vi "pyonpyon3.7.vi"() -> ()   [LabVIEW 2013]
uses:
  impl/CTL_pp3c_SessionParam.ctl
  impl/pp3_CTL_SessionInfo.ctl
  impl/CTL_pp3g_LoopState.ctl
  impl/pp3_CTL_BehavioralState.ctl
  impl/CTL_pp3g_Trial.ctl
  impl/pp3_CTL_TrialType.ctl
  labolabo2/waveforms/WFTypes.ctl
  impl/pp3_CTL_SessionParamDynamic.ctl
  impl/CTL_pp3c_DaqStatus.ctl
  <vilib>/userdefined/High Color/IMAQdx.ctl
  <vilib>/sound2/lvsound2.llb/Sound Output Task ID.ctl
  labolabo2/array/impl/NullArray_I.vi
  <vilib>/Utility/file.llb/Read From Spreadsheet File (string).vi
  labolabo2/array/impl/ArrayFirst_S.vi
panel:
  out "Session List Valid":bool=TRUE
  in  "Refresh info":bool
  in  "Session List Hidden":u8[](array[numeric])=[1, 1, 1, 2, 2, 2, 1, 1, 2, 2, 2, 1, 2, 1, 2, 2, 1, 1, 2, 2, 2, 1, 1, 1, 2, 2, 2, 1, 2, 1, 2, 1, 2, 1, 1, 1, 2, 2, 1, 2, 1, 1, 2, 1, 2, 1, 2, 1, 2, 2, 2, 1, 2, 1, 2, 1, 2, 1, 1, 1] min=1 step=1
  out "concatenated string":string="OS Name:                   Microsoft Wi\rOS Version:                6.1.7601 Service Pack 1 Build 7601\rSystem Type:               x64-based PC\rTime Zone:                 (UTC+01:00) Amsterdam, Berli\rTotal Physical Memory:     7,657 MB"
  out "Info VI Revision":string="1403" caption="Rev #"
  out "Info Hostname":string="PCR6985-17"
  out "Session list display":string[][](table)=[["1", "1", "1", "2", "2"], ["2", "1", "1", "2", "2"], ["2", "1", "2", "1", "2"], ["2", "1", "1", "2", "2"], ["2", "1", "1", "1", "2"], ["2", "2", "1", "2", "1"], ["2", "1", "2", "1", "1"], ["1", "2", "2", "1", "2"], ["1", "1", "2", "1", "2"], ["1", "2", "1", "2", "2"], ["2", "1", "2", "1", "2"], ["1", "2", "1", "1", "1"]]
  in  "Trial Types Control":enum32{"Trial Types Control"}(tab)
  out "Trial Types File Path":path=path "C:/Data/tDC.Coulb2/trial types/01_02__FM2k4k_4k2k.pp2tt.tsv"
  in  "Save Trial Types":bool
  in  "Load Trial Types":bool
  out "Trial Types Valid":bool=TRUE
  in  "Trial Types":T1[](array[typedef])=[{"Trial Type Number"=1, "Trial Type"=enum."GO", "Trial Weight"=1, "Shock (mA)"=-1.0, "Duration (ms)"=250.0, "Sound Type"=enum."04 FM Sweep", "Stim P1"=2000.0, "Stim P2"=4000.0, "Stim P3"=0.0, "Stim P4"=0.0, "DAQ Amplitude (V)"=1.0}, {"Trial Type Number"=2, "Trial Type"=enum."NOGO", "Trial Weight"=1, "Shock (mA)"=-1.0, "Duration (ms)"=250.0, "Sound Type"=enum."04 FM Sweep", "Stim P1"=4000.0, "Stim P2"=2000.0, "Stim P3"=0.0, "Stim P4"=0.0, "DAQ Amplitude (V)"=1.0}] {"DAQ Amplitude (V)" min=0.0 max=5.0 format="%_4g"; "Shock (mA)" min=-1.0 max=5.0; "Trial Weight" step=1; "Duration (ms)" min=0.0 max=1.0; "Trial Type Number" min=1 max=256 step=1}
  in  "Session List Control":enum32{"Session List Control"}(tab)
  out "Session List File Path":path
  in  "Load Session List":bool
  in  "Save Session List":bool
  in  "Generate Session List":bool
  in  "Total Trials":i32=60 min=3 max=122 step=1
  in  "Pseudo-Gell. Start":i32=2 min=0 max=3 step=1
  in  "60 trials":bool
  in  "90 trials":bool
  in  "test trials":bool
  in  "DAQ status variable":T4={"Sound AO"="Dev6/ao0", "Shock intesity AO"="Dev6/ao1", "Code_LED DO"="Dev6/port1:2", "Switch DI"="Dev6/port0/line0", "Webcam"="cam9", "Sound AO task"="", "Sound card task"=0, "Shock intensity AO task"="", "Code_LED DO task"="", "Switch DI task"="", "AO <=> Sound card"=FALSE, "Sound card"=0, "sample rate"=100000.0, "Variable shock"=TRUE, "Webcam on"=TRUE, "Waveform memo"={"t0"=timestamp(0 s since 1904-01-01), "dt"=1.0, "Y"=[]}, "Tone trigger"="PFI1", "Master-9 DO"="Dev6/port0/line5:7", "Master-9 DO task"="", "Master-9 on"=TRUE} caption="DAQ status variable  (initially to be read from /config/config.main.vi, change default settings there)" {"sample rate" min=8000.0; "Sound card task" format="%.0x"}
  out "Image":T7(plugin-control)
  in  "Session param (dynamic)":T8={"Def M shock (uA)"=720.0, "Def F shock (uA)"=150.0}
  in  "stop":bool
  in  "Pause":bool
  out "Loop state":T9={"Curr  tr"=2, "Curr (ms)"=2873456, "Cum (ms)"=46921, "Run loop diff"=11, "Tone countdown (ms)"=777777, "Countdown (ms)"=764, "Curr State"=enum."14 Intertrial Interval", "Prev State"=enum."9 NOGO Jumped", "Rw"=FALSE, "Sw"=FALSE, "Tone\nGate"=FALSE, "Punish"=FALSE, "Current DAQ DO Int"=0, "Current Loaded Trial"={"Trial Type Number"=2, "Trial Type"=enum."NOGO", "Trial Weight"=1, "Shock (mA)"=150.0, "Duration (ms)"=250.0, "Sound Type"=enum."04 FM Sweep", "Stim P1"=4000.0, "Stim P2"=2000.0, "Stim P3"=0.0, "Stim P4"=0.0, "DAQ Amplitude (V)"=1.0}, "Total trials memo"=60, "State start cum memo (ms)"=42685, "Last dur jump time memo (ms)"=1563, "Last dur shock time memo (ms)"=3019, "Tone repeat memo (ms)"=0, "Webcam on"=FALSE, "Webcam recording"=FALSE, "State update flag"=FALSE, "Last loaded shock voltage"=0.075, "Vid upd"=enum."0", "First time tone"=FALSE} {"Current DAQ DO Int" format="%016b"; "Current Loaded Trial"."DAQ Amplitude (V)" min=0.0 max=5.0 format="%_4g"; "Current Loaded Trial"."Shock (mA)" min=-1.0 max=5.0; "Current Loaded Trial"."Trial Weight" step=1; "Current Loaded Trial"."Duration (ms)" min=0.0 max=1.0; "Current Loaded Trial"."Trial Type Number" min=1 max=256 step=1}
  in  "Session parameters":T11={"Log File Directory Root"=path "E:/Data/SPP.Coulb1", "Subject Name"="test", "Tone repeat (ms)"=0, "Habit tr0 (s)"=180, "ITI min\n(s)"=14, "ITI max\n(s)"=24, "Stay \n(s)"=5, "Run"=FALSE, "Jump time\n(s)"=4, "Start trial"=0, "Log File Directory"=path "C:/Data/tDC.Coulb2/test/171120/163328", "Shock \ndur (s)"=6, "Pre click \n(V)"=0.1, "Click\ndel (s)"=1.0, "Reward CR"=FALSE} {"Click\ndel (s)" min=0.0 step=1.0; "Pre click \n(V)" min=0.0 max=1.0 step=1.0; "Shock \ndur (s)" min=0 step=1; "Stay \n(s)" min=0 step=1; "Start trial" step=1; "Jump time\n(s)" min=0 step=1; "Tone repeat (ms)" min=0 max=1000 step=1; "ITI min\n(s)" min=0 step=1; "ITI max\n(s)" min=0 step=1; "Habit tr0 (s)" min=0 step=1}
  out "Runtime Errors":errorcluster
  in  "Refresh":bool
  out "Session info":T12={"Total  Tr"=3, "G Tr"=2, "G Jump"=0, "G Jump%"=0.0, "N Tr"=1, "N Jump"=1, "N Jump%"=100.0, "T Tr"=0, "T Jump"=0, "T Jump%"=nan, "M shock dur (ms)"=1503.5, "F shock dur (ms)"=3019.0, "H latency (ms)"=0.0, "F latency (ms)"=1563.0, "T jump latency (ms)"=0.0} {"T Jump%" format="%.3g"; "N Jump%" format="%.3g"; "G Jump%" format="%.3g"}
  # "Pyonpyon Labview  v3.7 \n(2017.3 KT -- opto trig C)"
  # "60 trials:  180-14-24-5\n90 trials:  180-6-16-3"
  # "Code"
  # "Type"
  # "P 1"
  # "P 2"
  # "P 3"
  # "P 4 (opto)"
  # "Weight"
  # "Shock"
  # "Dur (ms)"
  # "DAQ Ampl (V)"
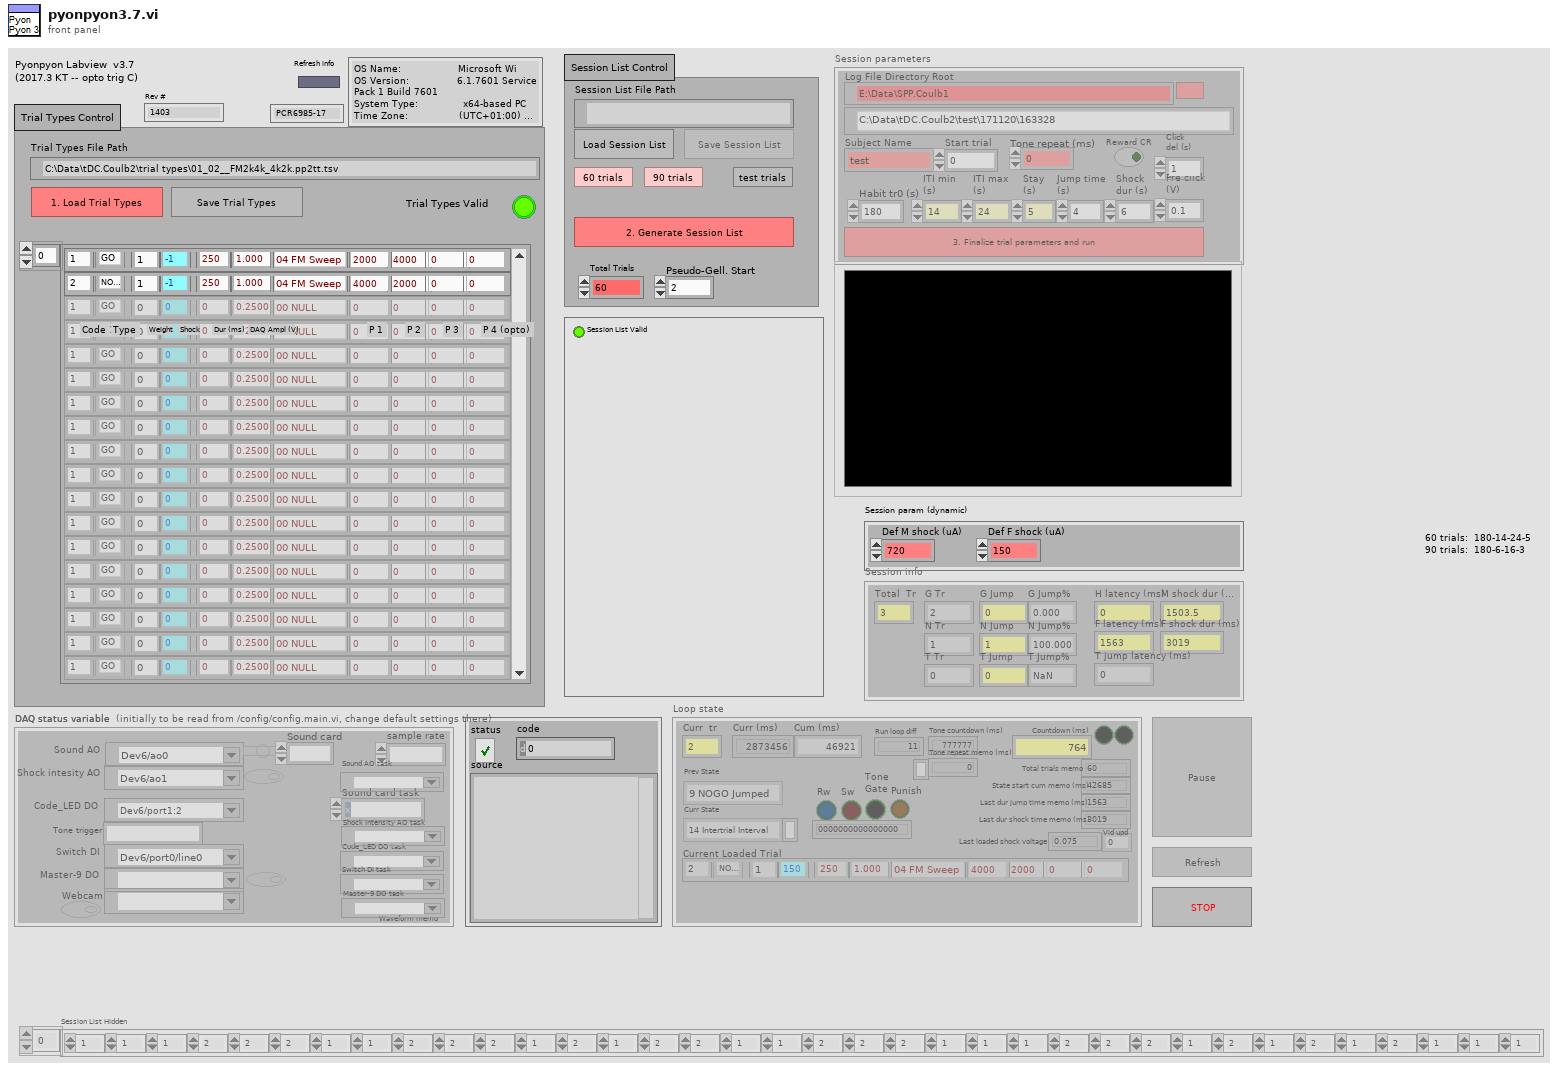
[diagram p1: front panel]
types:
  T1 = typedef "CTL_pp3g_Trial.ctl" = cluster{"Trial Type Number":i16, "Trial Type":T2, "Trial Weight":u32, "Shock (mA)":dbl, "Duration (ms)":dbl, "Sound Type":T3, "Stim P1":dbl, "Stim P2":dbl, "Stim P3":dbl, "Stim P4":dbl, "DAQ Amplitude (V)":dbl}
  T2 = typedef "pp3_CTL_TrialType.ctl" = enum16{"OFF", "GO", "NOGO", "TEST"}
  T3 = typedef "WFTypes.ctl" = enum16{"00 NULL", "01 DC", "02 Noise", "03 Pure Tone", "04 FM Sweep", "05 FM Sweep BURST"}
  T4 = typedef "CTL_pp3c_DaqStatus.ctl" = cluster{"Sound AO":tag, "Shock intesity AO":tag, "Code_LED DO":tag, "Switch DI":tag, "Webcam":T5, "Sound AO task":refnum<k21>, "Sound card task":T6, "Shock intensity AO task":refnum<k21>, "Code_LED DO task":refnum<k21>, "Switch DI task":refnum<k21>, "AO <=> Sound card":bool, "Sound card":u32, "sample rate":dbl, "Variable shock":bool, "Webcam on":bool, "Waveform memo":waveform(dbl), "Tone trigger":string, "Master-9 DO":tag, "Master-9 DO task":refnum<k21>, "Master-9 on":bool}
  T5 = typedef "IMAQdx.ctl" = refnum<k21>
  T6 = typedef "Sound Output Task ID.ctl" = u32
  T7 = typedef "IMAQ Image.ctl" = refnum<image>
  T8 = typedef "pp3_CTL_SessionParamDynamic.ctl" = cluster{"Def M shock (uA)":dbl, "Def F shock (uA)":dbl}
  T9 = typedef "CTL_pp3g_LoopState.ctl" = cluster{"Curr  tr":u16, "Curr (ms)":u32, "Cum (ms)":u64, "Run loop diff":i64, "Tone countdown (ms)":i64, "Countdown (ms)":i64, "Curr State":T10, "Prev State":T10, "Rw":bool, "Sw":bool, "Tone\nGate":bool, "Punish":bool, "Current DAQ DO Int":u16, "Current Loaded Trial":T1, "Total trials memo":i64, "State start cum memo (ms)":i64, "Last dur jump time memo (ms)":i64, "Last dur shock time memo (ms)":i64, "Tone repeat memo (ms)":i64, "Webcam on":bool, "Webcam recording":bool, "State update flag":bool, "Last loaded shock voltage":dbl, "Vid upd":enum16{"0", "1", "2", "3", "4", "5", "6", "7", "8", "9"}, "First time tone":bool}
  T10 = typedef "pp3_CTL_BehavioralState.ctl" = enum8{"0 NULL", "1 Habituation", "2 (Load Trial)", "3 Stay Period", "4 Load Audio/Click Delay", "5 GO Trial", "6 GO Jumped", "7 GO Timeout", "8 NOGO Trial", "9 NOGO Jumped", "10 NOGO Timeout", "11 TEST Trial", "12 TEST Jumped", "13 TEST Timeout", "14 Intertrial Interval", "15 Done"}
  T11 = typedef "CTL_pp3c_SessionParam.ctl" = cluster{"Log File Directory Root":path, "Subject Name":string, "Tone repeat (ms)":i32, "Habit tr0 (s)":i32, "ITI min\n(s)":i32, "ITI max\n(s)":i32, "Stay \n(s)":i32, "Run":bool, "Jump time\n(s)":i32, "Start trial":u16, "Log File Directory":path, "Shock \ndur (s)":i32, "Pre click \n(V)":dbl, "Click\ndel (s)":dbl, "Reward CR":bool}
  T12 = typedef "pp3_CTL_SessionInfo.ctl" = cluster{"Total  Tr":u32, "G Tr":u32, "G Jump":u32, "G Jump%":dbl, "N Tr":u32, "N Jump":u32, "N Jump%":dbl, "T Tr":u32, "T Jump":u32, "T Jump%":dbl, "M shock dur (ms)":dbl, "F shock dur (ms)":dbl, "H latency (ms)":dbl, "F latency (ms)":dbl, "T jump latency (ms)":dbl}
  T13 = enum8{"Enabled", "Disabled", "Disabled and Grayed Out"}
  T14 = enum16{"open", "replace", "create", "open or create", "replace or create", "replace or create with confirmation"}
  T15 = typedef "imagedata.ctl" = cluster{"image type":i32, "image depth":i32, "image":u8[], "mask":u8[], "colors":u32[], "Rectangle":cluster{"left":i16, "top":i16, "right":i16, "bottom":i16}}
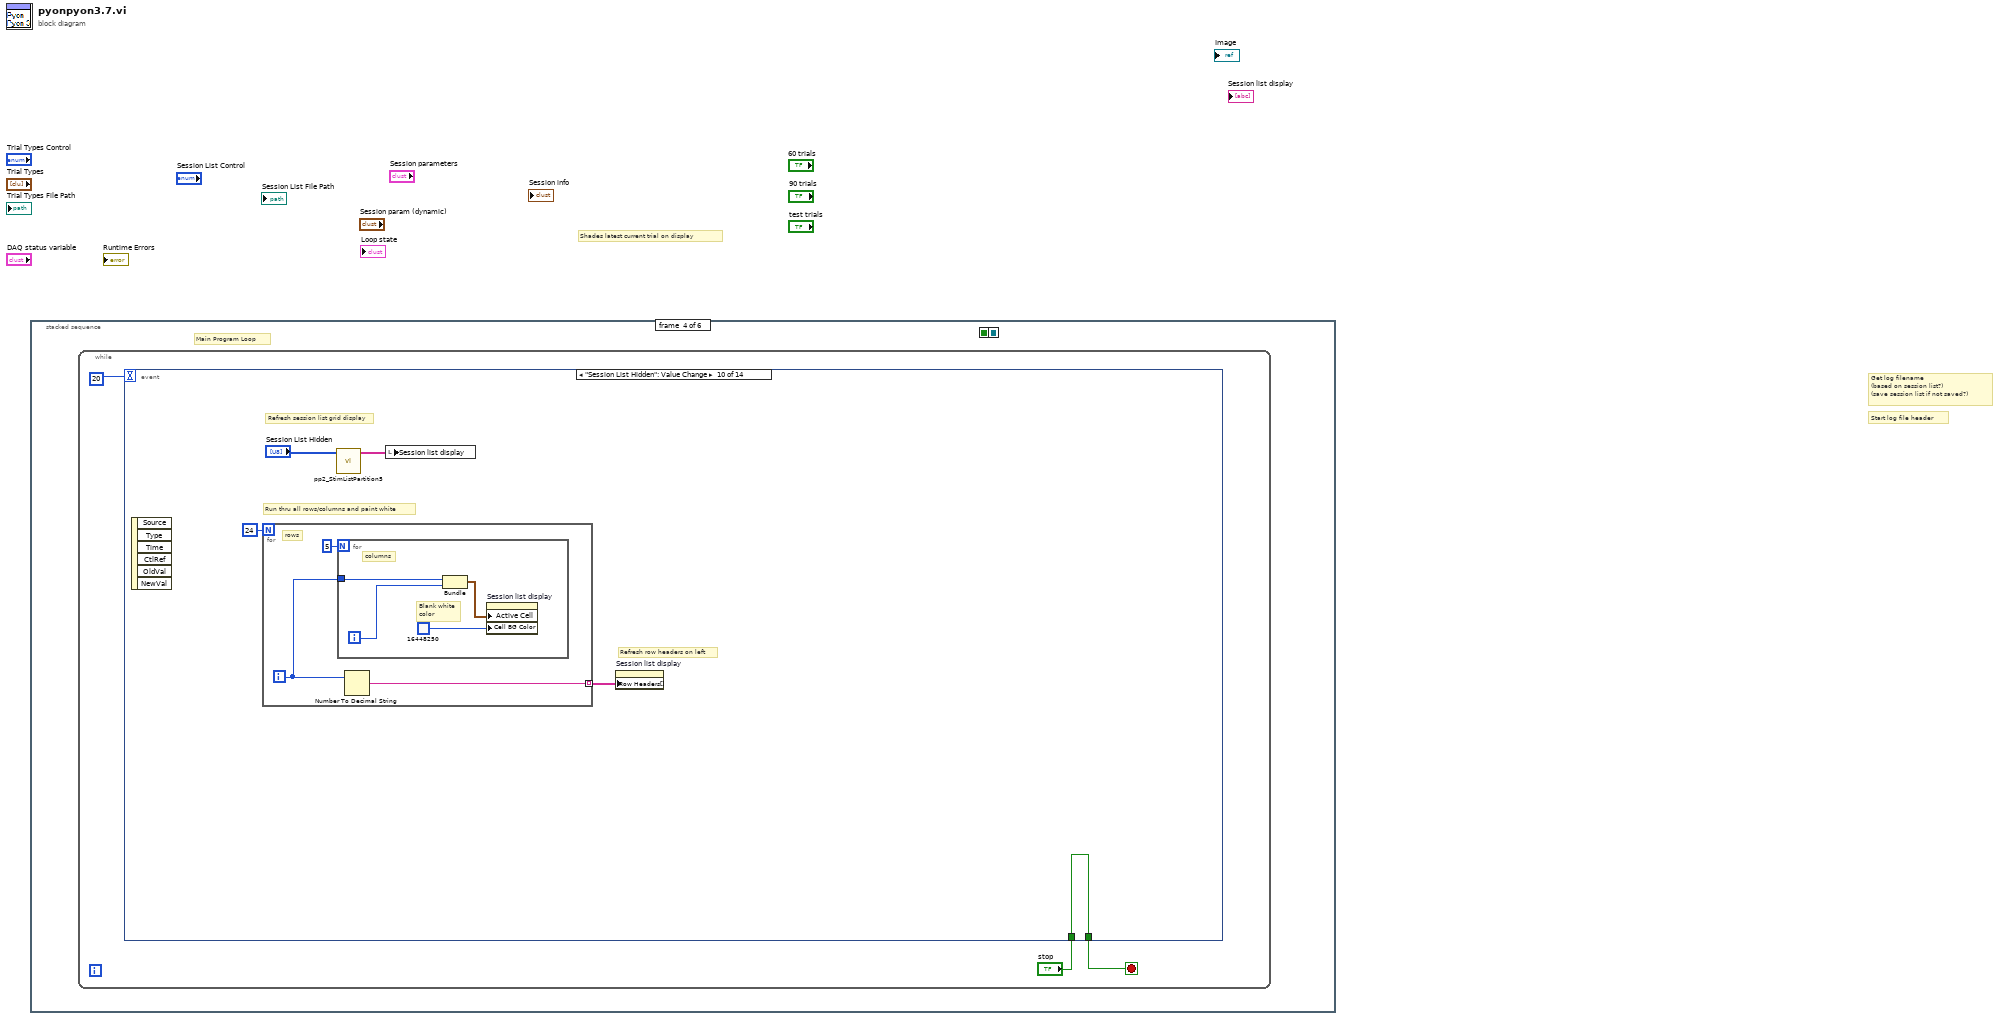
[diagram p0: block diagram]
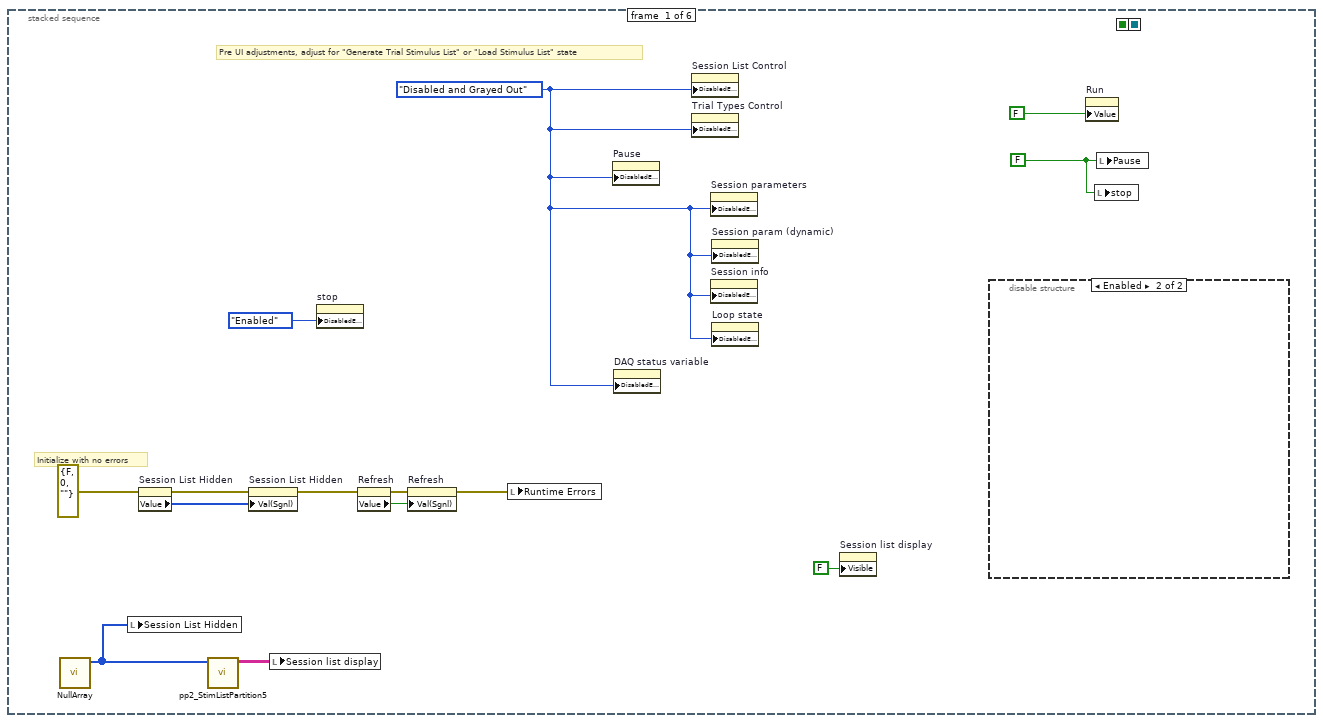
[diagram p2: hidden frame]
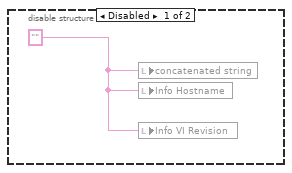
[diagram p3: hidden frame]
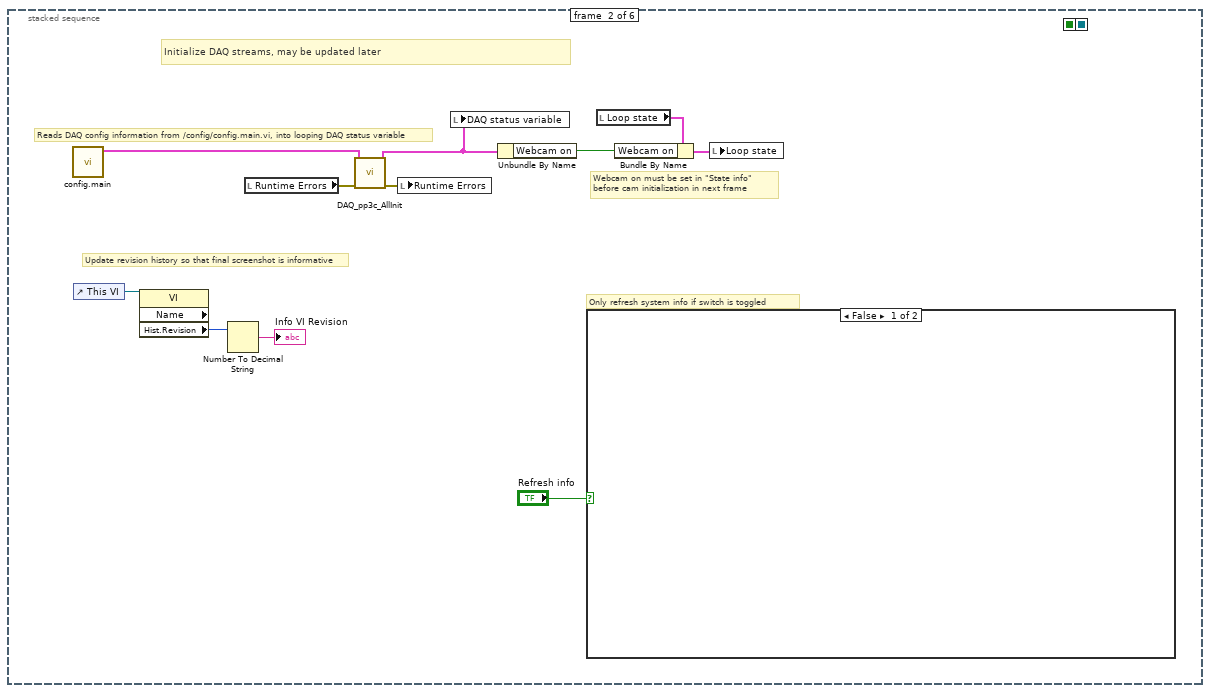
[diagram p4: hidden frame]
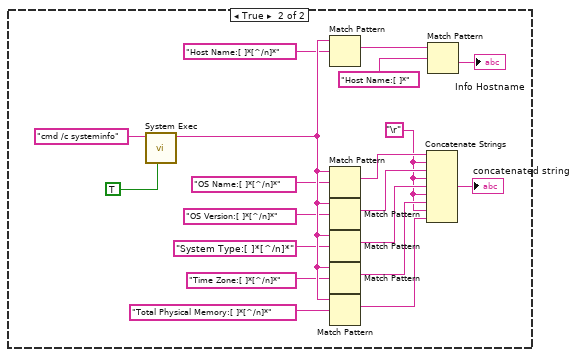
[diagram p5: hidden frame]
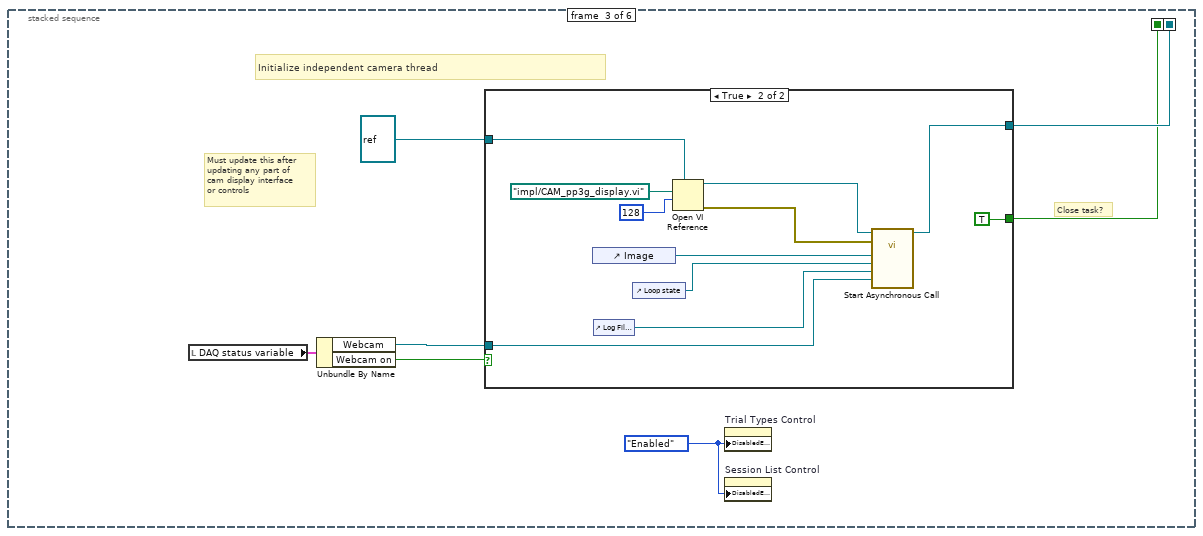
[diagram p6: hidden frame]
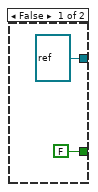
[diagram p7: hidden frame]
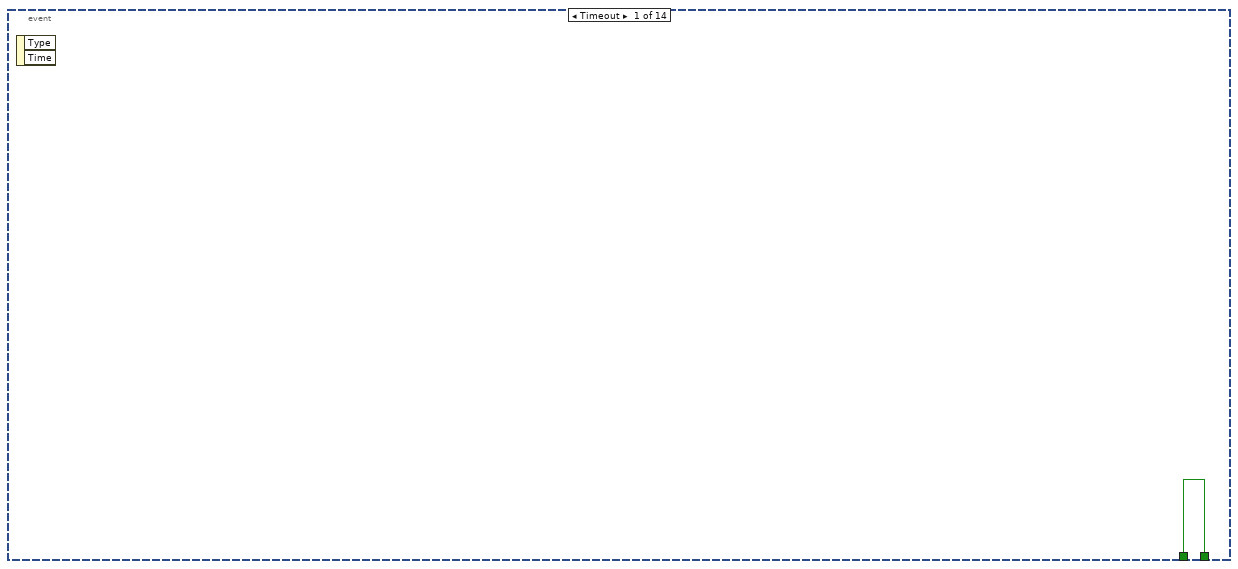
[diagram p8: hidden frame]
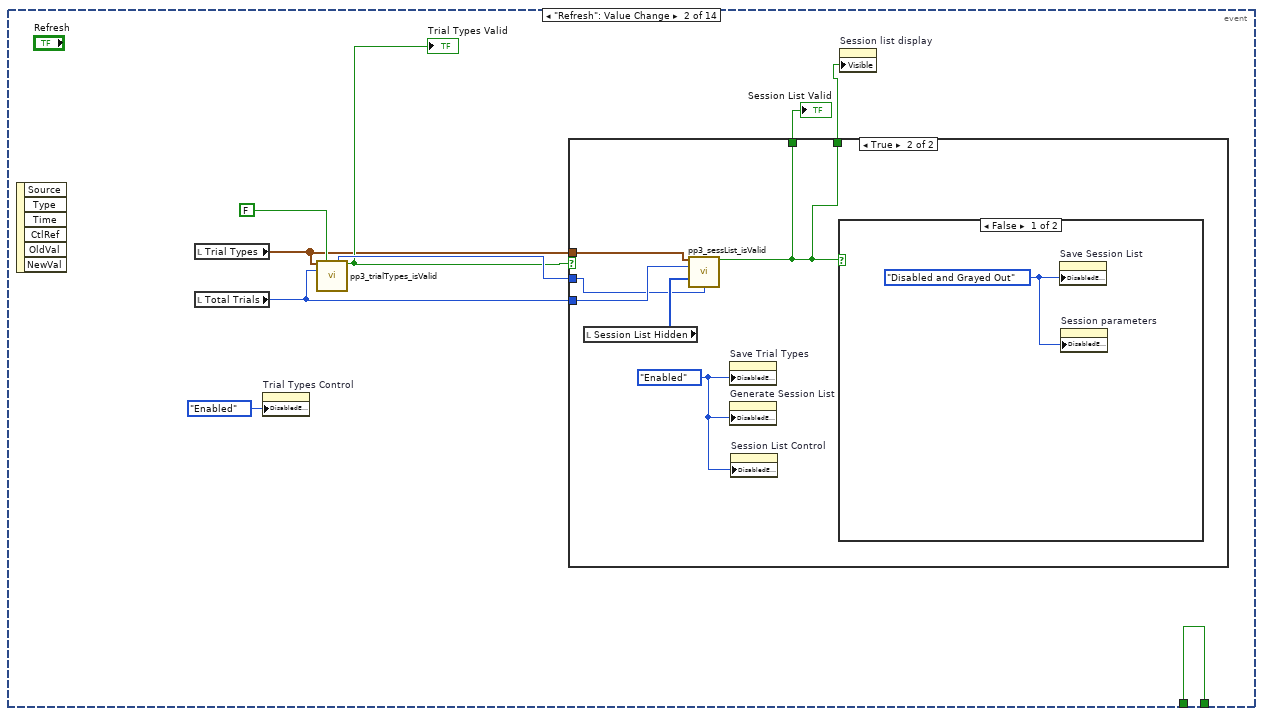
[diagram p9: hidden frame]
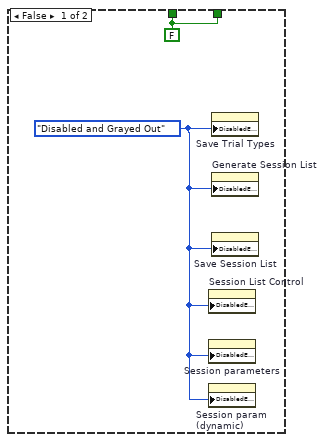
[diagram p10: hidden frame]
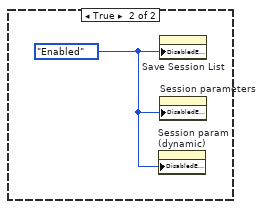
[diagram p11: hidden frame]
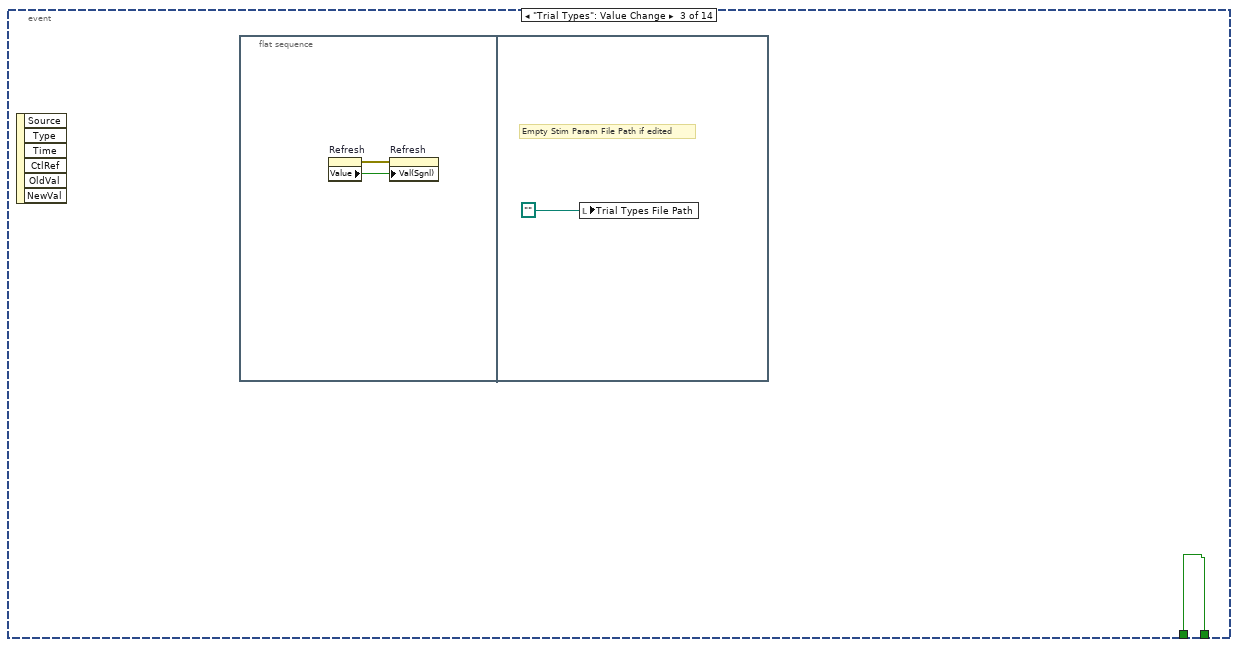
[diagram p12: hidden frame]
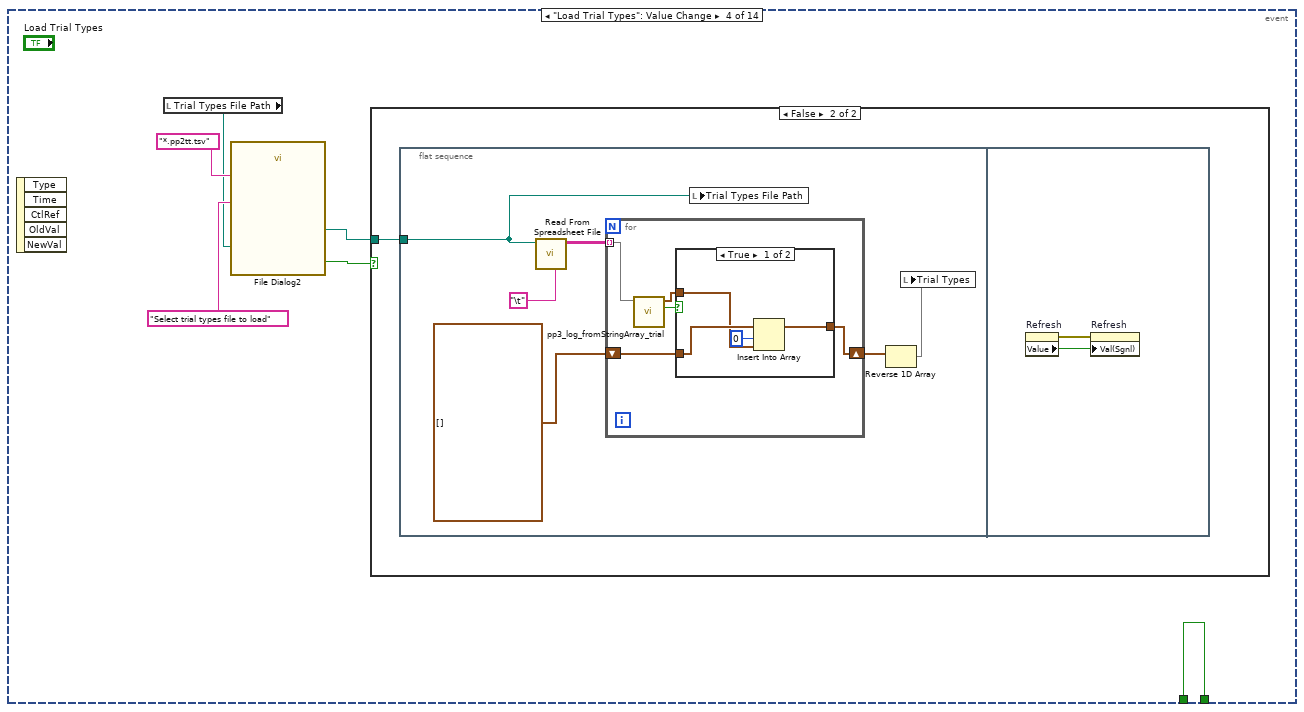
[diagram p13: hidden frame]
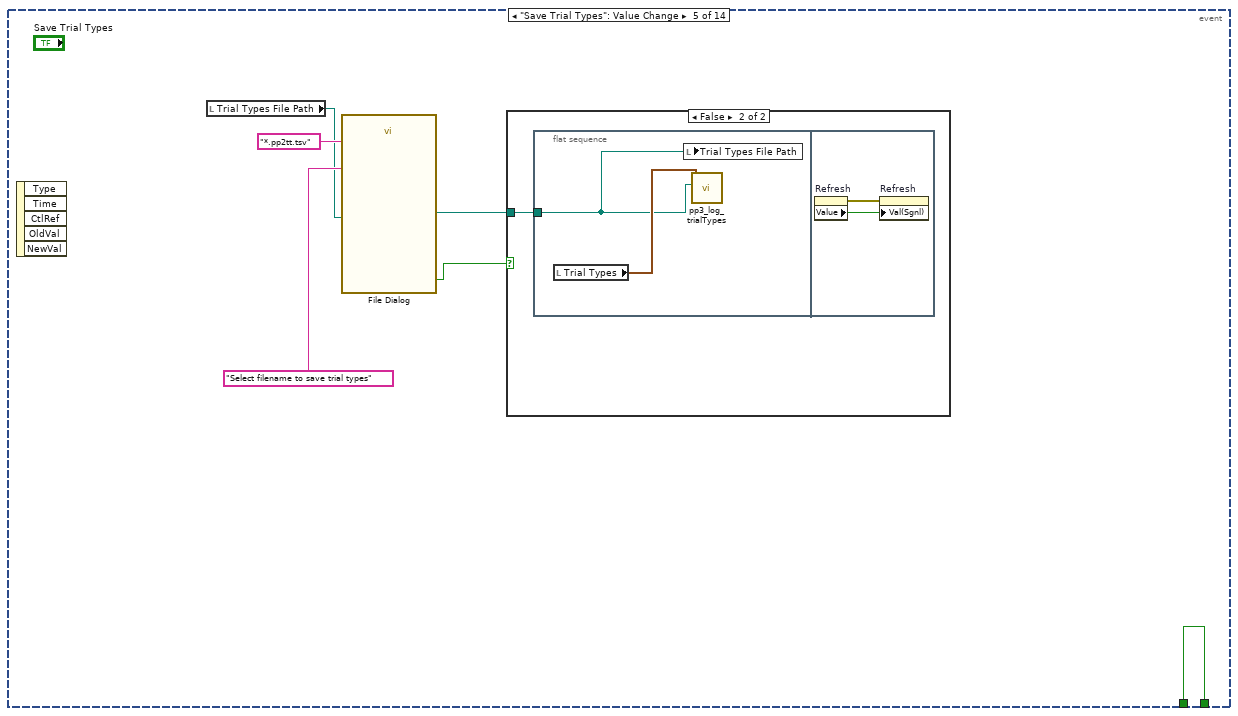
[diagram p16: hidden frame]
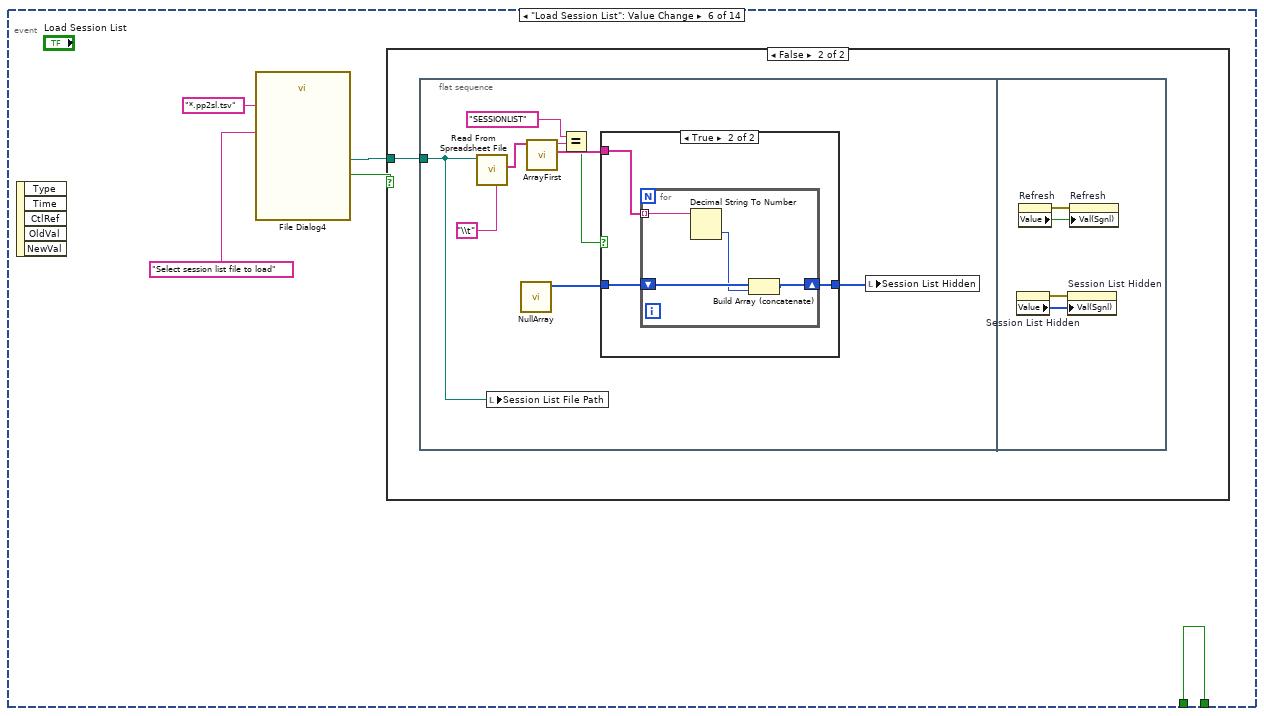
[diagram p18: hidden frame]
diagram:
  # "Shades latest current trial on display"
  # "Start log file header"
  # "Get log filename\n(based on session list?)\n(save session list if not saved?)"
  n1 = stacked-sequence {
    seq-local: [_ _ w49 _ _ _] -> [_ _ _ _ w731 _]
    seq-local: [_ _ w48 _ _ _] -> [_ _ _ _ w728 _]
    frame #0 {
      w14 = FALSE
      w1 = T13."Disabled and Grayed Out" ("Disabled")
      # "Initialize with no errors"
      # "Pre UI adjustments, adjust for \"Generate Trial Stimulus List\" or \"Load Stimulus List\" state"
      n2 = call-poly "NullArray.vi"() -> ("Null Array"=w5:i32[])  [unwired: 11 in]
      n3 = local write "Session List Hidden"(w5) -> ()
      n4 = property on="Session List Hidden" class="Arr (strict)"(error in=errorcluster {"status"=FALSE, "code"=0, "source"=""} ("error in (no error)")) -> (error out=w11:errorcluster, "Value"=w10:u8[])  [unwired: 1 in, 1 out]
      n5 = call "pp2_StimListPartition5.vi"("Session List (Hidden variable)"=w5) -> ("Session list display"=w4:string[][])  [unwired: 9 in]
      n6 = property on="Session List Hidden" class="Arr (strict)"(error in=w11, "Val(Sgnl)"=w10) -> (error out=w8:errorcluster)  [unwired: 1 in, 1 out]
      n7 = local write "Session list display"(w4) -> ()
      n8 = property on="stop" class="Bool (strict)"("DisabledEnum"=T13."Enabled" ("Disabled")) -> ()  [unwired: 2 in, 2 out]
      n9 = property on="Refresh" class="Bool (strict)"(error in=w8) -> (error out=w7:errorcluster, "Value"=w9:bool)  [unwired: 1 in, 1 out]
      n10 = property on="Refresh" class="Bool (strict)"(error in=w7, "Val(Sgnl)"=w9) -> (error out=w6:errorcluster)  [unwired: 1 in, 1 out]
      n11 = local write "Runtime Errors"(w6) -> ()
      n12 = property on="Pause" class="Bool (strict)"("DisabledEnum"=w1) -> ()  [unwired: 2 in, 2 out]
      n13 = property on="DAQ status variable" class="Clust (strict)"("DisabledEnum"=w1) -> ()  [unwired: 2 in, 2 out]
      n14 = property on="Session List Control" class="TabCtl (strict)"("DisabledEnum"=w1) -> ()  [unwired: 2 in, 2 out]
      n15 = property on="Trial Types Control" class="TabCtl (strict)"("DisabledEnum"=w1) -> ()  [unwired: 2 in, 2 out]
      n16 = property on="Session parameters" class="Clust (strict)"("DisabledEnum"=w1) -> ()  [unwired: 2 in, 2 out]
      n17 = property on="Session info" class="Clust (strict)"("DisabledEnum"=w1) -> ()  [unwired: 2 in, 2 out]
      n18 = property on="Session param (dynamic)" class="Clust (strict)"("DisabledEnum"=w1) -> ()  [unwired: 2 in, 2 out]
      n19 = property on="Loop state" class="Clust (strict)"("DisabledEnum"=w1) -> ()  [unwired: 2 in, 2 out]
      n20 = property on="Session list display" class="Tbl (strict)"("Visible"=FALSE) -> ()  [unwired: 2 in, 2 out]
      n21 = disable-structure shown="Enabled" {
        frame Disabled {
          w15 = "" ("concatenated string")
          n22 = local write "concatenated string"(w15) -> ()
          n23 = local write "Info Hostname"(w15) -> ()
          n24 = local write "Info VI Revision"(w15) -> ()
        }
        frame Enabled {
        }
      }
      n25 = property on="Run" class="Bool (strict)"("Value"=FALSE) -> ()  [unwired: 2 in, 2 out]
      n26 = local write "stop"(w14) -> ()
      n27 = local write "Pause"(w14) -> ()
    }
    frame #1 {
      # "Reads DAQ config information from /config/config.main.vi, into looping DAQ status variable"
      # "Update revision history so that final screenshot is informative"
      # "Only refresh system info if switch is toggled"
      # "Webcam on must be set in \"State info\"\nbefore cam initialization in next frame"
      # "Initialize DAQ streams, may be updated later"
      n28 = call "config.main.vi"() -> ("Daq status"=w16:T4)  [unwired: 11 in]
      n29 = control-ref of="This VI"() -> (w20:refnum<vi>)
      n30 = property class="VI" props=["Name", "Hist.Revision"](reference=w20) -> ("Hist.Revision"=w18:u32)  [unwired: 1 in, 3 out]
      n31 = Number To Decimal String(number=w18) -> (decimal integer string=→"Info VI Revision":string)  [unwired: 1 in]
      n32 = local read "Runtime Errors"() -> (w22:errorcluster)
      n33 = call "DAQ_pp3c_AllInit.vi"("error in (no error)"=w22, "Daq config in"=w16) -> ("error out"=w21:errorcluster, "Daq config out"=w26:T4)  [unwired: 8 in]
      n34 = local write "Runtime Errors"(w21) -> ()
      n35 = local write "DAQ status variable"(w26) -> ()
      n36 = Unbundle By Name(w26) -> ("Webcam on"=w24:bool)
      n37 = case shown="False" "Refresh info" {
        frame False {
        }
        frame True {
          w35 = "\r"
          n38 = call <vilib>:"System Exec.vi"("run minimized? (F)"=TRUE, "command line"="cmd /c systeminfo") -> ("standard output"=w34:string)  [unwired: 6 in, 3 out]
          n39 = Match Pattern(string=w34, regular expression="Host Name:[ ]*[^/n]*") -> (match substring=w27:string)  [unwired: 1 in, 3 out]
          n40 = Match Pattern(string=w34, regular expression="OS Name:[ ]*[^/n]*") -> (match substring=w41:string)  [unwired: 1 in, 3 out]
          n41 = Match Pattern(string=w34, regular expression="OS Version:[ ]*[^/n]*") -> (match substring=w40:string)  [unwired: 1 in, 3 out]
          n42 = Match Pattern(string=w34, regular expression="System Type:[ ]*[^/n]*") -> (match substring=w39:string)  [unwired: 1 in, 3 out]
          n43 = Match Pattern(string=w34, regular expression="Time Zone:[ ]*[^/n]*") -> (match substring=w38:string)  [unwired: 1 in, 3 out]
          n44 = Match Pattern(string=w34, regular expression="Total Physical Memory:[ ]*[^/n]*") -> (match substring=w37:string)  [unwired: 1 in, 3 out]
          n45 = Concatenate Strings(w41, w35, w40, w35, w39, w35, w38, w35, w37) -> (→"concatenated string":string)
          n46 = Match Pattern(string=w27, regular expression="Host Name:[ ]*") -> (after substring=→"Info Hostname":string)  [unwired: 1 in, 3 out]
        }
      }
      n47 = local read "Loop state"() -> (w25:T9)
      n48 = Bundle By Name(cluster=w25, "Webcam on"=w24) -> (w23:T9)
      n49 = local write "Loop state"(w23) -> ()
    }
    frame #2 {
      w47 = T13."Enabled" ("Disabled")
      # "Initialize independent camera thread"
      # "Close task?"
      # "Must update this after\nupdating any part of\ncam display interface\nor controls"
      n50 = local read "DAQ status variable"() -> (w51:T4)
      n51 = Unbundle By Name(w51) -> ("Webcam"=w52:T5, "Webcam on"=w50:bool)
      n52 = case shown="True" w50 {
        tunnel: w52 -> [_ w58]
        tunnel: [refnum<vi> refnum ("type specifier VI Refnum (for type only)") w62] -> w49
        tunnel: [FALSE TRUE] -> w48
        tunnel: refnum<vi> refnum ("type specifier VI Refnum (for type only)") -> [_ w57]
        frame False {
        }
        frame True {
          n53 = control-ref of="Image"() -> (w60:refnum<vi>)
          n54 = control-ref of="Log File Directory"() -> (w59:refnum<vi>)
          n55 = control-ref of="Loop state"() -> (w55:refnum<vi>)
          n56 = Open VI Reference(type specifier VI Refnum (for type only)=w57, vi path=path "impl/CAM_pp3g_display.vi", options=128) -> (vi reference=w56:refnum<vi>, error out=w61:errorcluster)  [unwired: 3 in]
          n57 = call-by-ref "Start Asynchronous Call"(reference=w56, error in=w61, "Camera"=w58, "Log File Directory"=w59, "Loop state Refnum"=w55, "Image Ctl Refnum"=w60) -> (reference out=w62:refnum<vi>)  [unwired: 8 in, 1 out]
        }
      }
      n58 = property on="Trial Types Control" class="TabCtl (strict)"("DisabledEnum"=w47) -> ()  [unwired: 2 in, 2 out]
      n59 = property on="Session List Control" class="TabCtl (strict)"("DisabledEnum"=w47) -> ()  [unwired: 2 in, 2 out]
    }
    frame #3 {
      # "Main Program Loop"
      n60 = while {
        stop <- w68 stop-if-true
        n61 = event shown="[9] \"Session List Hidden\": Value Change" {
          selector: _ -> [_ _ _ _ _ _ _ _ _ _ _ _ _ _]
          dyn-events: _ -> [_ _ _ _ _ _ _ _ _ _ _ _ _ _]
          timeout: u32 20 ("milliseconds to wait") -> [_ _ _ _ _ _ _ _ _ _ _ _ _ _]
          tunnel: [w69 w71 w89 w98 w123 w133 w156 w168 w192 w196 w208 w706 w713 w720] -> w68
          tunnel: "stop" -> [w69 w71 w89 w98 w123 w133 w156 w168 w192 w196 _ w706 w713 w720]
          event Timeout {
            n62 = event-data() -> ()  [unwired: 1 in, 2 out]
          }
          event "Refresh": Value Change {
            n63 = event-data() -> ()  [unwired: 1 in, 6 out]
            n64 = local read "Trial Types"() -> (w74:T1[])
            n65 = local read "Total Trials"() -> (w77:i32)
            n66 = property on="Trial Types Control" class="TabCtl (strict)"("DisabledEnum"=T13."Enabled" ("Disabled")) -> ()  [unwired: 2 in, 2 out]
            n67 = call "pp3_trialTypes_isValid.vi"("Trial Types In"=w74, "Throw Error"=FALSE, "Total Trials"=w77) -> ("Trial Replication Factor"=w78:i32, "Paradigm Valid?"=w75:bool)  [unwired: 7 in, 4 out]
            "Trial Types Valid" <- w75
            n68 = case shown="True" w75 {
              tunnel: w78 -> [_ w83]
              tunnel: w77 -> [_ w86]
              tunnel: w74 -> [_ w85]
              tunnel: [w79 w81] -> w73
              tunnel: [w79 w81] -> w70
              frame False {
                w79 = FALSE ("Session List Valid?")
                w80 = T13."Disabled and Grayed Out" ("Disabled")
                n69 = property on="Session List Control" class="TabCtl (strict)"("DisabledEnum"=w80) -> ()  [unwired: 2 in, 2 out]
                n70 = property on="Session parameters" class="Clust (strict)"("DisabledEnum"=w80) -> ()  [unwired: 2 in, 2 out]
                n71 = property on="Session param (dynamic)" class="Clust (strict)"("DisabledEnum"=w80) -> ()  [unwired: 2 in, 2 out]
                n72 = property on="Save Trial Types" class="Bool"("DisabledEnum"=w80) -> ()  [unwired: 2 in, 2 out]
                n73 = property on="Generate Session List" class="Bool"("DisabledEnum"=w80) -> ()  [unwired: 2 in, 2 out]
                n74 = property on="Save Session List" class="Bool"("DisabledEnum"=w80) -> ()  [unwired: 2 in, 2 out]
              }
              frame True {
                w82 = T13."Enabled" ("Disabled")
                n75 = local read "Session List Hidden"() -> (w84:u8[])
                n76 = call "pp3_sessList_isValid.vi"("Trial Types In"=w85, "Total Trials"=w86, "Session List"=w84, "Trial Replication Factor"=w83) -> ("Session List Valid?"=w81:bool)  [unwired: 11 in]
                n77 = property on="Save Trial Types" class="Bool"("DisabledEnum"=w82) -> ()  [unwired: 2 in, 2 out]
                n78 = property on="Generate Session List" class="Bool"("DisabledEnum"=w82) -> ()  [unwired: 2 in, 2 out]
                n79 = property on="Session List Control" class="TabCtl (strict)"("DisabledEnum"=w82) -> ()  [unwired: 2 in, 2 out]
                n80 = case shown="False" w81 {
                  frame False {
                    w87 = T13."Disabled and Grayed Out" ("Disabled")
                    n81 = property on="Save Session List" class="Bool"("DisabledEnum"=w87) -> ()  [unwired: 2 in, 2 out]
                    n82 = property on="Session parameters" class="Clust (strict)"("DisabledEnum"=w87) -> ()  [unwired: 2 in, 2 out]
                  }
                  frame True {
                    w88 = T13."Enabled" ("Disabled")
                    n83 = property on="Session param (dynamic)" class="Clust (strict)"("DisabledEnum"=w88) -> ()  [unwired: 2 in, 2 out]
                    n84 = property on="Save Session List" class="Bool"("DisabledEnum"=w88) -> ()  [unwired: 2 in, 2 out]
                    n85 = property on="Session parameters" class="Clust (strict)"("DisabledEnum"=w88) -> ()  [unwired: 2 in, 2 out]
                  }
                }
              }
            }
            "Session List Valid" <- w73
            n86 = property on="Session list display" class="Tbl (strict)"("Visible"=w70) -> ()  [unwired: 2 in, 2 out]
          }
          event "Trial Types": Value Change {
            n87 = event-data() -> ()  [unwired: 1 in, 6 out]
            n88 = flat-sequence {
              frame #0 {
                n89 = property on="Refresh" class="Bool (strict)"() -> (error out=w91:errorcluster, "Value"=w90:bool)  [unwired: 2 in, 1 out]
                n90 = property on="Refresh" class="Bool (strict)"(error in=w91, "Val(Sgnl)"=w90) -> ()  [unwired: 1 in, 2 out]
              }
              frame #1 {
                # "Empty Stim Param File Path if edited"
                n91 = local write "Trial Types File Path"(path "") -> ()
              }
            }
          }
          event "Load Trial Types": Value Change {
            n92 = event-data() -> ()  [unwired: 1 in, 5 out]
            n93 = local read "Trial Types File Path"() -> (w93:path)
            n94 = call "File Dialog2"("start path"=w93, "prompt"="Select trial types file to load", "pattern (all files)"="*.pp2tt.tsv") -> ("selected path"=w95:path, "cancelled"=w94:bool)  [unwired: 9 in, 2 out]
            n95 = case shown="False" w94 {
              tunnel: w95 -> [_ w99]
              frame True {
              }
              frame False {
                n96 = flat-sequence {
                  tunnel: w99 -> [w101]
                  frame #0 {
                    n97 = call-poly <vilib>:"Read From Spreadsheet File.vi"("delimiter (\\t)"="\t" ("delimiter (\\t)"), "file path (dialog if empty)"=w101) -> ("all rows"=w105:string[][])  [unwired: 5 in, 4 out]
                    n98 = for {
                      tunnel: w105 -> [w109] mode=indexing
                      shift-right: [w107] -> w103
                      shift-left: T1[] [] -> [w108]
                      n99 = call "pp3_log_fromStringArray_trial.vi"("Input string array"=w109) -> ("Was TRIAL?"=w106:bool, "Trial in"=w110:T1)  [unwired: 7 in]
                      n100 = case shown="True" w106 {
                        tunnel: w110 -> [w113 _]
                        tunnel: w108 -> [w114 w115]
                        tunnel: [w111 w115] -> w107
                        frame True {
                          n101 = Insert Into Array(array=w114, index=0, new element=w113) -> (w111:T1[])
                        }
                        frame False {
                        }
                      }
                    }
                    n102 = local write "Trial Types File Path"(w101) -> ()
                    n103 = Reverse 1D Array(array=w103) -> (reversed array=w102:T1[])
                    n104 = local write "Trial Types"(w102) -> ()
                  }
                  frame #1 {
                    n105 = property on="Refresh" class="Bool (strict)"() -> (error out=w117:errorcluster, "Value"=w116:bool)  [unwired: 2 in, 1 out]
                    n106 = property on="Refresh" class="Bool (strict)"(error in=w117, "Val(Sgnl)"=w116) -> ()  [unwired: 1 in, 2 out]
                  }
                }
              }
            }
          }
          event "Save Trial Types": Value Change {
            n107 = event-data() -> ()  [unwired: 1 in, 5 out]
            n108 = local read "Trial Types File Path"() -> (w119:path)
            n109 = call "File Dialog"("start path"=w119, "prompt"="Select filename to save trial types", "pattern (all files)"="*.pp2tt.tsv") -> ("selected path"=w120:path, "cancelled"=w118:bool)  [unwired: 9 in, 2 out]
            n110 = case shown="False" w118 {
              tunnel: w120 -> [_ w124]
              frame True {
              }
              frame False {
                n111 = flat-sequence {
                  tunnel: w124 -> [w125]
                  frame #0 {
                    n112 = local read "Trial Types"() -> (w126:T1[])
                    n113 = local write "Trial Types File Path"(w125) -> ()
                    n114 = call "pp3_log_trialTypes.vi"("Trial Types File Path"=w125, "Trial Types"=w126) -> ()  [unwired: 10 in]
                  }
                  frame #1 {
                    n115 = property on="Refresh" class="Bool (strict)"() -> (error out=w127:errorcluster, "Value"=w128:bool)  [unwired: 2 in, 1 out]
                    n116 = property on="Refresh" class="Bool (strict)"(error in=w127, "Val(Sgnl)"=w128) -> ()  [unwired: 1 in, 2 out]
                  }
                }
              }
            }
          }
          event "Load Session List": Value Change {
            n117 = event-data() -> ()  [unwired: 1 in, 5 out]
            n118 = call "File Dialog4"("prompt"="Select session list file to load", "pattern (all files)"="*.pp2sl.tsv") -> ("selected path"=w130:path, "cancelled"=w129:bool)  [unwired: 10 in, 2 out]
            n119 = case shown="False" w129 {
              tunnel: w130 -> [_ w134]
              frame True {
              }
              frame False {
                n120 = flat-sequence {
                  tunnel: w134 -> [w138]
                  frame #0 {
                    n121 = call-poly <vilib>:"Read From Spreadsheet File.vi"("delimiter (\\t)"="\\t" ("delimiter (\\t)"), "file path (dialog if empty)"=w138) -> ("first row"=w142:string[])  [unwired: 5 in, 4 out]
                    n122 = local write "Session List File Path"(w138) -> ()
                    n123 = call-poly "NullArray.vi"() -> ("Null Array"=w135:i32[])  [unwired: 11 in]
                    n124 = call-poly "ArrayFirst.vi"("1D Array In"=w142) -> ("Rest of Array"=w139:string[], "First Element"=w141:string)  [unwired: 9 in]
                    n125 = Equal?(x="SESSIONLIST", y=w141) -> (x = y?=w137:bool)
                    n126 = case shown="True" w137 {
                      tunnel: w139 -> [_ w147]
                      tunnel: [w144 w146] -> w136
                      tunnel: w135 -> [w144 w145]
                      frame False {
                      }
                      frame True {
                        n127 = for {
                          shift-right: [w151] -> w146
                          shift-left: w145 -> [w150]
                          tunnel: w147 -> [w149] mode=indexing
                          n128 = Decimal String To Number(string=w149) -> (number=w148:i32)  [unwired: 2 in, 1 out]
                          n129 = Build Array (concatenate)(w150, w148) -> (w151:i32[])
                        }
                      }
                    }
                    n130 = local write "Session List Hidden"(w136) -> ()
                  }
                  frame #1 {
                    n131 = property on="Session List Hidden" class="Arr (strict)"() -> (error out=w152:errorcluster, "Value"=w153:u8[])  [unwired: 2 in, 1 out]
                    n132 = property on="Refresh" class="Bool (strict)"() -> (error out=w155:errorcluster, "Value"=w154:bool)  [unwired: 2 in, 1 out]
                    n133 = property on="Session List Hidden" class="Arr (strict)"(error in=w152, "Val(Sgnl)"=w153) -> ()  [unwired: 1 in, 2 out]
                    n134 = property on="Refresh" class="Bool (strict)"(error in=w155, "Val(Sgnl)"=w154) -> ()  [unwired: 1 in, 2 out]
                  }
                }
              }
            }
          }
          event "Save Session List": Value Change {
            n135 = event-data() -> ()  [unwired: 1 in, 5 out]
            n136 = flat-sequence {
              frame #0 {
                n137 = call "File Dialog3"("prompt"="Select filename to save session list", "pattern (all files)"="*.pp2sl.tsv") -> ("selected path"=w160:path, "cancelled"=w159:bool)  [unwired: 10 in, 2 out]
                n138 = case shown="False" w159 {
                  tunnel: w160 -> [_ w163]
                  frame True {
                  }
                  frame False {
                    n139 = local read "Session List Hidden"() -> (w165:u8[])
                    n140 = call "pp2_log_toString_sessionList.vi"("Session List in"=w165) -> ("spreadsheet string"=w164:string)  [unwired: 10 in]
                    n141 = Write to Text File(file (use dialog)=w163, text=w164) -> (refnum out=w161:refnum<file>, error out=w162:errorcluster)  [unwired: 2 in, 1 out]
                    n142 = Close File(refnum=w161, error in=w162) -> ()  [unwired: 2 out]
                    n143 = local write "Session List File Path"(w163) -> ()
                  }
                }
              }
              frame #1 {
                n144 = property on="Refresh" class="Bool (strict)"() -> (error out=w167:errorcluster, "Value"=w166:bool)  [unwired: 2 in, 1 out]
                n145 = property on="Refresh" class="Bool (strict)"(error in=w167, "Val(Sgnl)"=w166) -> ()  [unwired: 1 in, 2 out]
              }
            }
          }
          event "Generate Session List": Value Change {
            n146 = event-data() -> ()  [unwired: 1 in, 5 out]
            n147 = flat-sequence {
              frame #0 {
                # "Empty file name if generating list"
                n148 = local read "Trial Types"() -> (w175:T1[])
                n149 = local read "Total Trials"() -> (w169:i32)
                n150 = Array Size(array=w175) -> (size(s)=w174:i32)
                n151 = Equal?(x=w174, y=1) -> (x = y?=w172:bool)
                n152 = case shown="False" w172 {
                  tunnel: w175 -> [w181 w184]
                  tunnel: [w176 w183] -> w170
                  tunnel: w169 -> [w177 w182]
                  frame True {
                    # "If only one trial type, just\nrepetitions of that trial in a row"
                    n153 = Index Array(array=w181, index=0) -> (element=w179:T1)
                    n154 = Unbundle By Name(w179) -> ("Trial Type Number"=w178:i16)
                    n155 = Initialize Array(w178, w177) -> (w176:i16[])
                  }
                  frame False {
                    n156 = call "pp3_sessList_createPseudoGellerman.vi"("Start Num"="Pseudo-Gell. Start", "Total Trials"=w182, "Trial Types"=w184) -> ("Session List (Cannot Edit)"=w183:i32[])  [unwired: 7 in, 1 out]
                  }
                }
                n157 = local write "Session List File Path"(path "") -> ()
                n158 = local write "Session List Hidden"(w170) -> ()
              }
              frame #1 {
                n159 = property on="Session List Hidden" class="Arr (strict)"() -> (error out=w187:errorcluster, "Value"=w186:u8[])  [unwired: 2 in, 1 out]
                n160 = property on="Session list display" class="Tbl (strict)"() -> (error out=w189:errorcluster, "Value"=w188:string[][])  [unwired: 2 in, 1 out]
                n161 = property on="Refresh" class="Bool (strict)"() -> (error out=w191:errorcluster, "Value"=w190:bool)  [unwired: 2 in, 1 out]
                n162 = property on="Session list display" class="Tbl (strict)"(error in=w189, "Val(Sgnl)"=w188) -> ()  [unwired: 1 in, 2 out]
                n163 = property on="Refresh" class="Bool (strict)"(error in=w191, "Val(Sgnl)"=w190) -> ()  [unwired: 1 in, 2 out]
                n164 = property on="Session List Hidden" class="Arr (strict)"(error in=w187, "Val(Sgnl)"=w186) -> ()  [unwired: 1 in, 2 out]
              }
            }
          }
          event "Total Trials": Value Change {
            n165 = event-data() -> ()  [unwired: 1 in, 6 out]
            n166 = flat-sequence {
              tunnel: "Total Trials" -> [_]
              frame #0 {
              }
              frame #1 {
                n167 = property on="Refresh" class="Bool (strict)"() -> (error out=w194:errorcluster, "Value"=w195:bool)  [unwired: 2 in, 1 out]
                n168 = property on="Refresh" class="Bool (strict)"(error in=w194, "Val(Sgnl)"=w195) -> ()  [unwired: 1 in, 2 out]
              }
            }
          }
          event "Session List Hidden": Value Change {
            # "Run thru all rows/columns and paint white"
            # "Refresh row headers on left"
            # "Refresh session list grid display"
            n169 = event-data() -> ()  [unwired: 1 in, 6 out]
            n170 = for {
              N: 24 -> [_]
              tunnel: [w201] -> w197 mode=indexing
              i -> [w202]
              # "rows"
              n171 = for {
                N: 5 -> [_]
                tunnel: w202 -> [w207]
                i -> [w206]
                # "columns"
                # "Blank white\ncolor"
                n172 = Bundle(w207, w206) -> (w205:cluster{i32, i32})  [unwired: 1 in]
                n173 = property on="Session list display" class="Tbl (strict)"("Active Cell"=w205, "Cell BG Color"=u32 16448250) -> ()  [unwired: 2 in, 2 out]
              }
              n174 = Number To Decimal String(number=w202) -> (decimal integer string=w201:string)  [unwired: 1 in]
            }
            n175 = call "pp2_StimListPartition5.vi"("Session List (Hidden variable)"="Session List Hidden") -> ("Session list display"=w199:string[][])  [unwired: 9 in]
            n176 = local write "Session list display"(w199) -> ()
            n177 = property on="Session list display" class="Tbl (strict)"("Row Headers[]"=w197) -> ()  [unwired: 2 in, 2 out]
          }
          event Value Change {
            # "Log Que"
            n178 = event-data() -> ()  [unwired: 1 in, 6 out]
            n179 = stacked-sequence {
              seq-local: [_ _ w281 _ _ _] -> [_ _ _ w331 _ _]
              seq-local: [_ _ _ w339 _ _] -> [_ _ _ _ w694 _]
              seq-local: [_ _ _ w329 _ _] -> [_ _ _ _ w693 _]
              tunnel: [_ _ _ w330 _ _] -> w208
              frame #0 {
                w209 = T13."Disabled" ("Disabled")
                w210 = T13."Disabled and Grayed Out" ("Disabled")
                # "Confirm if starting with nonzero trial"
                # "GUI Adjustments (pre)"
                n180 = local read "Session parameters"() -> (w211:T11)
                n181 = flat-sequence {
                  tunnel: w210 -> [w215]
                  frame #0 {
                    n182 = property on="Session List Control" class="TabCtl (strict)"("DisabledEnum"=w215) -> ()  [unwired: 2 in, 2 out]
                  }
                  frame #1 {
                    n183 = property on="Session list display" class="Tbl (strict)"("DisabledEnum"=T13."Disabled" ("Disabled")) -> ()  [unwired: 2 in, 2 out]
                  }
                }
                n184 = Unbundle By Name(w211) -> ("Start trial"=w212:u16)
                n185 = property on="Trial Types Control" class="TabCtl (strict)"("DisabledEnum"=w210) -> ()  [unwired: 2 in, 2 out]
                n186 = property on="Session parameters" class="Clust (strict)"("DisabledEnum"=w210) -> ()  [unwired: 2 in, 2 out]
                n187 = Not Equal To 0?(x=w212) -> (x != 0?=w213:bool)
                n188 = case shown="True" w213 {
                  tunnel: w212 -> [_ w220]
                  tunnel: w211 -> [_ w217]
                  frame False {
                  }
                  frame True {
                    n189 = Number To Decimal String(number=w220) -> (decimal integer string=w221:string)  [unwired: 1 in]
                    n190 = Concatenate Strings("Really start with nonzero trial?: " ("message"), w221) -> (w219:string)
                    n191 = Two Button Dialog(message=w219, 1:"No, start from zero" ("F button name (\"Cancel\")"), 2:"Yes" ("T button name (\"OK\")")) -> (T button?=w218:bool)
                    n192 = case shown="False" w218 {
                      tunnel: w217 -> [w227 _]
                      frame False {
                        n193 = Bundle By Name(cluster=w227, "Start trial"=u16 0) -> (w225:T11)
                        n194 = local write "Session parameters"(w225) -> ()
                      }
                      frame True {
                        # "Just proceed"
                      }
                    }
                  }
                }
                n195 = disable-structure shown="Disabled" {
                  frame Disabled {
                    n196 = property on="Pause" class="Bool (strict)"("DisabledEnum"=T13."Enabled" ("Disabled")) -> ()  [unwired: 2 in, 2 out]
                  }
                  frame Enabled {
                  }
                }
                n197 = property on="Loop state" class="Clust (strict)"("DisabledEnum"=w209) -> ()  [unwired: 2 in, 2 out]
                n198 = property on="Session info" class="Clust (strict)"("DisabledEnum"=w209) -> ()  [unwired: 2 in, 2 out]
              }
              frame #1 {
                # "ToDo... go through\nsequence for starting\nat trial !=0 for new\nlog, when state info is not\ninitialized yet!"
                # "If webcam is on, start recording"
                # "Reset trial to zero if exceeded total"
                # "If starting from trial zero, clear and habituate, if not, directly to load trial"
                # "Pre-behavior state and statistics adjustments"
                n199 = local read "Session parameters"() -> (w246:T11)
                n200 = Unbundle By Name(w246) -> ("Start trial"=w241:u16, "Habit tr0 (s)"=w229:i32, "Tone repeat (ms)"=w237:i32, "Reward CR"=w228:bool)
                n201 = local read "Session List Hidden"() -> (w239:u8[])
                n202 = Array Size(array=w239) -> (size(s)=w238:i32)
                n203 = Greater Than 0?(x=w229) -> (x > 0?=w232:bool)
                n204 = Greater Or Equal?(x=w241, y=w238) -> (x >= y?=w242:bool)
                n205 = case shown="True" w242 {
                  tunnel: w241 -> [w260 _]
                  tunnel: [w260 u16 0 ("Curr  tr")] -> w240
                  frame False {
                  }
                  frame True {
                  }
                }
                n206 = Equal To 0?(x=w240) -> (x = 0?=w230:bool)
                n207 = And(x=w230, y=w232) -> (x .and. y?=w231:bool)
                n208 = local read "Loop state"() -> (w236:T9)
                n209 = Unbundle By Name(w236) -> ("Webcam on"=w235:bool)
                n210 = Bundle By Name(cluster=w236, "Curr  tr"=w240, "Curr State"=pp3_CTL_BehavioralState."1 Habituation", "Prev State"=pp3_CTL_BehavioralState."0 NULL", "Total trials memo"=w238, "Tone repeat memo (ms)"=w237, "Webcam recording"=w235) -> (w243:T9)
                n211 = case shown="True" w230 {
                  tunnel: w243 -> [w262 w269]
                  tunnel: w229 -> [_ _]
                  tunnel: [w262 w263] -> w234
                  frame False {
                  }
                  frame True {
                    # "Reset time and info only\nif for 0th trial????!!!"
                    n212 = Tick Count (ms)() -> (millisecond timer value=w268:u32)
                    n213 = To Quad Integer(1:w268) -> (0:w267:i64)
                    n214 = Bundle By Name(cluster=w269, "Curr (ms)"=w267, "Cum (ms)"=i64 0) -> (w263:T9)
                    n215 = local read "Session info"() -> (w264:T12)
                    n216 = call "pp2_updateSessionInfoCLEAR.vi"("Session info In"=w264) -> ("Session info Out"=w265:T12)  [unwired: 10 in]
                    n217 = local write "Session info"(w265) -> ()
                  }
                }
                n218 = case shown="True" w231 {
                  tunnel: w234 -> [w248 w255]
                  tunnel: [w249 w254] -> w233
                  tunnel: w229 -> [_ w253]
                  tunnel: w228 -> [w247 w252]
                  frame False {
                    n219 = call "LOOP_pp3c_NextState.vi"("Reward CR"=w247, "New state countdown (ms)"=i64 0, "New State"=pp3_CTL_BehavioralState."2 (Load Trial)", "State In"=w248) -> ("State Out"=w249:T9)  [unwired: 7 in]
                  }
                  frame True {
                    # "Habituation only if 0th trial and habituation length >0"
                    n220 = To Quad Integer(1:w253) -> (0:w256:i64)
                    n221 = Multiply(x=w256, y=i64 1000) -> (x*y=w257:i64)
                    n222 = call "LOOP_pp3c_NextState.vi"("Reward CR"=w252, "New state countdown (ms)"=w257, "New State"=pp3_CTL_BehavioralState."1 Habituation", "State In"=w255) -> ("State Out"=w254:T9)  [unwired: 7 in]
                  }
                }
                n223 = local write "Loop state"(w233) -> ()
              }
              frame #2 {
                w288 = "\t"
                # "Serialize DAQ configurations for logging que"
                # "Initialize logging queues and log directory"
                n224 = Get Date/Time In Seconds() -> (seconds since 1Jan1904=w305:timestamp)
                n225 = local read "Session parameters"() -> (w317:T11)
                n226 = Obtain Queue(name (unnamed)="RL Log Queue", element data type="") -> (queue out=w272:refnum<queue>)  [unwired: 3 in, 2 out]
                n227 = Unbundle By Name(w317) -> ("Log File Directory Root"=w304:path, "Subject Name"=w315:string)
                n228 = Format Date/Time String(time format string (%c)="\\%y%m%d\\%H%M%S\\", seconds (now)=w305) -> (date/time string=w316:string)  [unwired: 1 in]
                n229 = Format Date/Time String(time format string (%c)="%y%m%d_%H%M%S.pp2tt.tsv" ("pattern (all files)"), seconds (now)=w305) -> (date/time string=w313:string)  [unwired: 1 in]
                n230 = Format Date/Time String(time format string (%c)="%y%m%d_%H%M%S.pp2sl.tsv" ("pattern (all files)"), seconds (now)=w305) -> (date/time string=w307:string)  [unwired: 1 in]
                n231 = Format Date/Time String(time format string (%c)="%y%m%d_%H%M%S.pp2rl.tsv" ("pattern (all files)"), seconds (now)=w305) -> (date/time string=w303:string)  [unwired: 1 in]
                n232 = Open VI Reference(type specifier VI Refnum (for type only)=refnum<vi> refnum, vi path=path "C:/Packages/pyonpyon/LV2/impl/pp2_log_SpawnRLLogger.vi", options=128) -> (vi reference=w277:refnum<vi>, error out=w276:errorcluster)  [unwired: 3 in]
                n233 = Concatenate Strings(w315, w316) -> (w314:string)
                n234 = Build Path(base path=w304, name or relative path=w314) -> (appended path=w296:path)
                n235 = Create Folder(path (use dialog)=w296) -> (created path=w290:path)  [unwired: 2 in, 2 out]
                n236 = disable-structure shown="Disabled" {
                  disable-tunnel: w313 -> [w321 _]
                  disable-tunnel: w290 -> [w318 _]
                  frame Disabled {
                    (unwired) TRUE ("Actually Run?")
                    n237 = Build Path(base path=w318, name or relative path=w321) -> (appended path=w320:path)
                    n238 = local read "Trial Types"() -> (w319:T1[])
                    n239 = call "pp3_log_trialTypes.vi"("Trial Types File Path"=w320, "Trial Types"=w319) -> ()  [unwired: 10 in]
                  }
                  frame Enabled {
                  }
                }
                n240 = Build Path(base path=w290, name or relative path=w303) -> (appended path=w273:path)
                n241 = call-by-ref "Start Asynchronous Call"(reference=w277, error in=w276, "file path in"=w273, "queue in"=w272) -> ()  [unwired: 10 in, 2 out]
                n242 = Build Path(base path=w290, name or relative path=w307) -> (appended path=w298:path)
                n243 = local read "Session List Hidden"() -> (w309:u8[])
                n244 = Bundle By Name(cluster=w317, "Log File Directory"=w290) -> (w270:T11)
                n245 = local read "DAQ status variable"() -> (w312:T4)
                n246 = Build Path(base path=w290, name or relative path="cam\\") -> (appended path=w294:path)
                n247 = local read "Info Hostname"() -> (w287:string)
                n248 = local read "Info VI Revision"() -> (w286:string)
                n249 = Create Folder(path (use dialog)=w294) -> ()  [unwired: 2 in, 3 out]
                n250 = call "pp3b_log_DAQconfig.vi"("queue in"=w272, "Daq config"=w312) -> ("queue out"=w284:refnum<queue>)  [unwired: 9 in]
                n251 = call "pp2_log_toString_sessionList.vi"("Session List in"=w309) -> ("spreadsheet string"=w308:string)  [unwired: 10 in]
                n252 = local write "Session parameters"(w270) -> ()
                n253 = call "pp3_log_sessionParameters.vi"("queue in"=w284) -> ("queue out"=w292:refnum<queue>)  [unwired: 10 in]
                n254 = Open/Create/Replace File(file path (use dialog)=w298, operation (0:open)=T14."create") -> (refnum out=w299:refnum<file>)  [unwired: 4 in, 2 out]
                n255 = call "pp3_log_trialMemo.vi"("queue in"=w292) -> ("queue out"=w293:refnum<queue>)  [unwired: 10 in]
                n256 = Concatenate Strings("RUNLOG" ("string"), w288, w287, w288, " " ("string"), w288, w286, "\r") -> (w282:string)
                n257 = call "LOG_pp3c_STATE.vi"("Log memo?"=TRUE, "queue in"=w293) -> ("queue out"=w283:refnum<queue>)  [unwired: 9 in]
                n258 = Write to Text File(file (use dialog)=w299, text=w308) -> (refnum out=w310:refnum<file>, error out=w311:errorcluster)  [unwired: 2 in, 1 out]
                n259 = Close File(refnum=w310, error in=w311) -> ()  [unwired: 2 out]
                n260 = Enqueue Element(queue=w283, element=w282) -> (queue out=w281:refnum<queue>)  [unwired: 2 in, 2 out]
              }
              frame #3 {
                w322 = 1000 ("y")
                # "Stop whole VI if \"Stop\" pushed or end reached"
                # "Main Behavior Loop"
                n261 = local read "Session parameters"() -> (w353:T11)
                n262 = Unbundle By Name(w353) -> ("ITI max\n(s)"=w343:i32, "ITI min\n(s)"=w342:i32, "Stay \n(s)"=w326:i32, "Jump time\n(s)"=w325:i32, "Shock \ndur (s)"=w324:i32, "Pre click \n(V)"=w347:dbl, "Click\ndel (s)"=w323:dbl, "Reward CR"=w328:bool)
                n263 = local read "DAQ status variable"() -> (w337:T4)
                n264 = local read "Loop state"() -> (w333:T9)
                n265 = local read "Session info"() -> (w332:T12)
                n266 = local read "Runtime Errors"() -> (w338:errorcluster)
                n267 = Multiply(x=w322, y=w343) -> (x*y=w345:i32)
                n268 = Multiply(x=w322, y=w342) -> (x*y=w344:i32)
                n269 = Multiply(x=w322, y=w326) -> (x*y=w354:i32)
                n270 = Multiply(x=w322, y=w325) -> (x*y=w351:i32)
                n271 = Multiply(x=w322, y=w324) -> (x*y=w350:i32)
                n272 = Multiply(x=w322, y=w323) -> (x*y=w336:dbl)
                n273 = To Quad Integer(1:w350) -> (0:w348:i64)
                n274 = To Quad Integer(1:w345) -> (0:w341:i64)
                n275 = To Quad Integer(1:w344) -> (0:w340:i64)
                n276 = To Quad Integer(1:w354) -> (0:w352:i64)
                n277 = To Quad Integer(1:w351) -> (0:w349:i64)
                n278 = To Quad Integer(1:w336) -> (0:w335:i64)
                n279 = while {
                  shift-right: [w384] -> w334
                  shift-left: w333 -> [w383]
                  shift-right: [w382] -> _
                  shift-left: w332 -> [w387]
                  shift-right: [w367] -> w329
                  shift-left: w331 -> [w361]
                  tunnel: w352 -> [w381]
                  tunnel: w349 -> [w380]
                  tunnel: w348 -> [w379]
                  tunnel: w347 -> [w378]
                  shift-right: [w377] -> w339
                  shift-left: w338 -> [w371]
                  shift-right: [w375] -> _
                  shift-left: FALSE -> [w376]
                  tunnel: w341 -> [w374]
                  tunnel: w340 -> [w373]
                  tunnel: w335 -> [w368]
                  tunnel: [w364] -> w330
                  tunnel: w328 -> [w358]
                  shift-right: [w357] -> w327
                  shift-left: w337 -> [w356]
                  stop <- w370 stop-if-true
                  # "Reward CR\n(only relevant for entering 6/10)"
                  # "Update display"
                  # "Update error display here"
                  # "Pre click (V)"
                  # "Click del (ms)"
                  # "Jump time (ms)"
                  # "Stay (ms)"
                  # "ITI max/min (ms)"
                  # "Shock dur (ms)"
                  # "Done and timed out"
                  # "Exitable?"
                  # "Once marker\n(reset to False automatically\nat loop end for most types)"
                  # "State timeout?"
                  # "Side changed?"
                  n280 = call "LOOP_pp3d_updateSideState.vi"("error in (no error)"=w371, "log queue in"=w361, "Daq config In"=w356, "State In"=w383) -> ("error out"=w355:errorcluster, "log queue out"=w360:refnum<queue>, "State Out"=w359:T9, "State timeout"=w386:bool, "Side change"=w385:bool)  [unwired: 3 in]
                  n281 = local write "Runtime Errors"(w371) -> ()
                  n282 = local write "Loop state"(w359) -> ()
                  n283 = Unbundle By Name(w359) -> ("Curr State"=w369:T10)
                  n284 = case shown="\"4 Load Audio/Click Delay\"" w369 {
                    selector: w369 -> [_ _ _ _ w515 _ _ _ _]
                    tunnel: w387 -> [w397 w419 w436 w485 w521 w586 w617 w636 w689]
                    tunnel: w359 -> [w399 w411 w440 w477 w525 w590 w621 w637 w688]
                    tunnel: w386 -> [w391 _ w437 w483 w523 w589 _ w641 w686]
                    tunnel: w385 -> [_ _ w441 _ w526 w588 _ _ _]
                    tunnel: [w398 w423 w439 w486 w524 w593 w620 w640 w688] -> w384
                    tunnel: [w397 w419 w436 w485 w521 w586 w617 w635 w689] -> w382
                    tunnel: w381 -> [_ w420 w438 _ _ _ _ _ _]
                    tunnel: w380 -> [_ _ _ w487 _ _ _ _ _]
                    tunnel: w379 -> [_ _ _ _ w522 _ _ _ _]
                    tunnel: w378 -> [_ _ w431 _ _ _ _ _ _]
                    tunnel: w355 -> [w395 w418 w435 w479 w519 w582 w616 w632 w690]
                    tunnel: [w395 w417 w434 w478 w518 w581 w616 w631 w690] -> w377
                    tunnel: w376 -> [_ _ _ w481 _ _ _ w639 w691]
                    tunnel: [FALSE FALSE FALSE w480 FALSE FALSE FALSE w638 w691] -> w375
                    tunnel: w374 -> [_ _ _ _ _ w592 w623 _ _]
                    tunnel: w373 -> [_ _ _ _ _ w591 w622 _ _]
                    tunnel: [TRUE FALSE FALSE FALSE FALSE FALSE FALSE TRUE TRUE] -> w372
                    tunnel: w368 -> [_ _ w430 _ _ _ _ _ _]
                    tunnel: w360 -> [w392 w409 w429 w482 w516 w584 w614 w633 w687]
                    tunnel: [w392 w408 w429 w482 w516 w584 w614 w633 w687] -> w367
                    tunnel: [FALSE ("State timeout") FALSE ("State timeout") FALSE ("State timeout") FALSE ("State timeout") FALSE ("State timeout") FALSE ("State timeout") FALSE ("State timeout") FALSE ("State timeout") w686] -> w362
                    tunnel: w358 -> [w389 w407 w427 w474 w513 w580 w612 _ _]
                    tunnel: [w388 w406 w426 w473 w511 w579 w611 w626 w684] -> w357
                    tunnel: w356 -> [w388 w406 w425 w472 w512 w578 w611 w627 w684]
                    frame "1 Habituation" {
                      n285 = case shown="True" w391 {
                        tunnel: w399 -> [w400 w405]
                        tunnel: [w400 w404] -> w398
                        tunnel: w389 -> [_ w401]
                        frame False {
                        }
                        frame True {
                          # "Load next if timeout"
                          n286 = call "LOOP_pp3c_NextState.vi"("Reward CR"=w401, "New state countdown (ms)"=i64 0, "New State"=pp3_CTL_BehavioralState."2 (Load Trial)", "State In"=w405) -> ("State Out"=w404:T9)  [unwired: 7 in]
                        }
                      }
                      n287 = Wait Until Next ms Multiple(millisecond multiple=u32 3) -> ()  [unwired: 1 out]
                    }
                    frame "2 (Load Trial)" {
                      # "Load curr trial and apply variable shock if on.\n(will not increment)"
                      n288 = local read "Session param (dynamic)"() -> (w414:T8)
                      n289 = local read "Session List Hidden"() -> (w415:u8[])
                      n290 = local read "Trial Types"() -> (w416:T1[])
                      n291 = disable-structure shown="Disabled" {
                        frame Disabled {
                          n292 = Wait Until Next ms Multiple(millisecond multiple=u32 1) -> ()  [unwired: 1 out]
                        }
                        frame Enabled {
                        }
                      }
                      n293 = call "LOOP_pp3c_loadNextTrial.vi"("State Info In"=w411, "Session param (dynamic)"=w414, "Session List (Hidden variable)"=w415, "Trial Types"=w416, "Daq config In"=w406, "log queue in"=w409, "error in (no error)"=w418) -> ("State Info Out"=w422:T9, "log queue out"=w408:refnum<queue>, "error out"=w417:errorcluster)  [unwired: 6 in]
                      n294 = call "LOOP_pp3c_NextState.vi"("Reward CR"=w407, "New state countdown (ms)"=w420, "New State"=pp3_CTL_BehavioralState."3 Stay Period", "State In"=w422) -> ("State Out"=w423:T9)  [unwired: 7 in]
                    }
                    frame "3 Stay Period" {
                      n295 = case shown="False" w441 {
                        tunnel: w440 -> [w452 w471]
                        tunnel: [w447 w470] -> w439
                        tunnel: w438 -> [_ w468]
                        tunnel: w437 -> [w451 _]
                        tunnel: w435 -> [w450 w467]
                        tunnel: [w449 w467] -> w434
                        tunnel: [w448 w465] -> w426
                        tunnel: w431 -> [w446 _]
                        tunnel: w430 -> [w445 _]
                        tunnel: w427 -> [w444 w466]
                        tunnel: w425 -> [w443 w465]
                        frame False {
                          n296 = case shown="True" w451 {
                            tunnel: w452 -> [w455 w464]
                            tunnel: w450 -> [w454 w462]
                            tunnel: [w454 w461] -> w449
                            tunnel: [w453 w456] -> w448
                            tunnel: [w455 w460] -> w447
                            tunnel: w446 -> [_ w459]
                            tunnel: w445 -> [_ w458]
                            tunnel: w444 -> [_ w457]
                            tunnel: w443 -> [w453 w456]
                            frame False {
                              # "No side change, no timeout"
                            }
                            frame True {
                              # "If stay timed out without side change, \ntrigger change to (Load audio) and play click"
                              n297 = call "LOOP_pp3c_NextState.vi"("Reward CR"=w457, "New state countdown (ms)"=w458, "New State"=pp3_CTL_BehavioralState."4 Load Audio/Click Delay", "State In"=w464) -> ("State Out"=w460:T9)  [unwired: 7 in]
                              n298 = call "DAQ_pp3c_AudioPlayClick.vi"("State In"=w460, "Daq config"=w456, "Pre click \n(V)"=w459, "error in (no error)"=w462) -> ("error out"=w461:errorcluster)  [unwired: 6 in]
                            }
                          }
                        }
                        frame True {
                          # "If side changed during stay, reload stay period\n(will not log state change, 3 == 3)"
                          n299 = call "LOOP_pp3c_NextState.vi"("Reward CR"=w466, "New state countdown (ms)"=w468, "New State"=pp3_CTL_BehavioralState."3 Stay Period", "State In"=w471) -> ("State Out"=w470:T9)  [unwired: 7 in]
                        }
                      }
                      n300 = disable-structure shown="Disabled" {
                        frame Disabled {
                          n301 = Wait Until Next ms Multiple(millisecond multiple=u32 1) -> ()  [unwired: 1 out]
                        }
                        frame Enabled {
                        }
                      }
                    }
                    frame "4 Load Audio/Click Delay" {
                      n302 = case shown="False" w481 {
                        selector: w481 -> [_ w499]
                        tunnel: [TRUE w499] -> w480
                        tunnel: w479 -> [w495 w500]
                        tunnel: [w494 w497] -> w473
                        tunnel: [w493 w500] -> w478
                        tunnel: w477 -> [w492 w498]
                        tunnel: [w490 w498] -> w476
                        tunnel: w472 -> [w489 w497]
                        frame False {
                          # "Load audio just once"
                          n303 = call "LOOP_pp3c_AudioLoadWaveform.vi"("State Info In"=w492, "Daq config In"=w489, "error in (no error)"=w495) -> ("Daq config Out"=w494:T4, "error out"=w493:errorcluster)  [unwired: 11 in]
                          n304 = Bundle By Name(cluster=w492, "Tone countdown (ms)"=i64 0) -> (w490:T9)
                        }
                        frame True {
                          # "has already happend once"
                        }
                      }
                      n305 = case shown="True" w483 {
                        tunnel: w487 -> [_ w505]
                        tunnel: [w501 w506] -> w486
                        tunnel: w476 -> [w501 w503]
                        tunnel: w474 -> [_ w502]
                        frame False {
                        }
                        frame True {
                          n306 = Unbundle By Name(w503) -> ("Current Loaded Trial.Trial Type"=w507:T2)
                          n307 = case shown="\"TEST\", Default" w507 {
                            tunnel: [pp3_CTL_BehavioralState."5 GO Trial" ("New State") pp3_CTL_BehavioralState."11 TEST Trial" ("New State") pp3_CTL_BehavioralState."8 NOGO Trial" ("New State")] -> w504
                            frame "GO" {
                            }
                            frame "TEST", Default {
                            }
                            frame "NOGO" {
                            }
                          }
                          n308 = call "LOOP_pp3c_NextState.vi"("Reward CR"=w502, "New state countdown (ms)"=w505, "New State"=w504, "State In"=w503) -> ("State Out"=w506:T9)  [unwired: 7 in]
                        }
                      }
                      n309 = disable-structure shown="Disabled" {
                        frame Disabled {
                          n310 = Wait Until Next ms Multiple(millisecond multiple=u32 1) -> ()  [unwired: 1 out]
                        }
                        frame Enabled {
                        }
                      }
                    }
                    frame "5 GO Trial", "8 NOGO Trial", "11 TEST Trial" {
                      n311 = case shown="False" w526 {
                        tunnel: w525 -> [w536 w567]
                        tunnel: [w535 w569] -> w524
                        tunnel: w523 -> [w537 _]
                        tunnel: w522 -> [w534 w563]
                        tunnel: [w533 w561] -> w511
                        tunnel: w519 -> [w532 w568]
                        tunnel: [w531 w568] -> w518
                        tunnel: w515 -> [w530 w566]
                        tunnel: w513 -> [w529 w562]
                        tunnel: w512 -> [w528 w561]
                        frame False {
                          n312 = case shown="False" w537 {
                            tunnel: w536 -> [w540 w552]
                            tunnel: [w539 w551] -> w535
                            tunnel: w534 -> [_ w547]
                            tunnel: [w543 w544] -> w533
                            tunnel: w532 -> [w542 w550]
                            tunnel: [w541 w550] -> w531
                            tunnel: w530 -> [_ w546]
                            tunnel: w529 -> [_ w545]
                            tunnel: w528 -> [w538 w544]
                            frame False {
                              # "continue/start  sound,\nretrigger if necessary"
                              n313 = call "DAQ_pp3c_AudioRetriggerDelayConditioning.vi"("Daq config In"=w538, "State In"=w540, "error in (no error)"=w542) -> ("Daq config Out"=w543:T4, "State Out"=w539:T9, "error out"=w541:errorcluster)  [unwired: 10 in]
                            }
                            frame True {
                              n314 = case shown="Default" w546 {
                                selector: w546 -> [w554 _ _ _]
                                tunnel: [w554 pp3_CTL_BehavioralState."7 GO Timeout" ("New State") pp3_CTL_BehavioralState."10 NOGO Timeout" ("New State") pp3_CTL_BehavioralState."13 TEST Timeout" ("New State")] -> w549
                                tunnel: [i64 0 ("New state countdown (ms)") w555 i64 0 ("New state countdown (ms)") i64 0 ("New state countdown (ms)")] -> w548
                                tunnel: w547 -> [_ w555 _ _]
                                frame Default {
                                # "Will not happen"
                                }
                                frame "5 GO Trial" {
                                # "If timout, miss!!!"
                                }
                                frame "8 NOGO Trial" {
                                # "If time out,\ncorrect rejection!!!"
                                }
                                frame "11 TEST Trial" {
                                }
                              }
                              n315 = call "LOOP_pp3c_NextState.vi"("Reward CR"=w545, "New state countdown (ms)"=w548, "New State"=w549, "State In"=w552) -> ("State Out"=w551:T9)  [unwired: 7 in]
                            }
                          }
                        }
                        frame True {
                          n316 = case shown="\"5 GO Trial\"" w566 {
                            selector: w566 -> [w571 _ _ _]
                            tunnel: [w571 pp3_CTL_BehavioralState."6 GO Jumped" ("New State") pp3_CTL_BehavioralState."9 NOGO Jumped" ("New State") pp3_CTL_BehavioralState."12 TEST Jumped" ("New State")] -> w564
                            tunnel: [i64 0 ("New state countdown (ms)") i64 0 ("New state countdown (ms)") w574 i64 0 ("New state countdown (ms)")] -> w565
                            tunnel: w563 -> [_ _ w574 _]
                            frame Default {
                              # "Will not happen"
                            }
                            frame "5 GO Trial" {
                              # "If side changed, hit!!!"
                            }
                            frame "8 NOGO Trial" {
                              # "If side changed,\nfalse alarm!!!"
                            }
                            frame "11 TEST Trial" {
                              # "If side changed, hit!!!"
                            }
                          }
                          n317 = call "LOOP_pp3c_NextState.vi"("Reward CR"=w562, "New state countdown (ms)"=w565, "New State"=w564, "State In"=w567) -> ("State Out"=w569:T9)  [unwired: 7 in]
                        }
                      }
                      n318 = disable-structure shown="Disabled" {
                        frame Disabled {
                          n319 = Wait Until Next ms Multiple(millisecond multiple=u32 1) -> ()  [unwired: 1 out]
                        }
                        frame Enabled {
                        }
                      }
                    }
                    frame "7 GO Timeout", "9 NOGO Jumped" {
                      # "Shock end should be ASAP"
                      n320 = Or(x=w588, y=w589) -> (x .or. y?=w587:bool)
                      n321 = case shown="True" w587 {
                        tunnel: [w597 w609] -> w593
                        tunnel: w592 -> [_ w608]
                        tunnel: w591 -> [_ w607]
                        tunnel: w590 -> [w598 w605]
                        tunnel: [w601 w602] -> w579
                        tunnel: w582 -> [w600 w604]
                        tunnel: [w599 w604] -> w581
                        tunnel: w580 -> [_ w603]
                        tunnel: w578 -> [w596 w602]
                        frame False {
                          # "continue/start  sound,\nretrigger if necessary"
                          # "Continue shock"
                          n322 = call "DAQ_pp3c_AudioRetriggerDelayConditioning.vi"("Daq config In"=w596, "State In"=w598, "error in (no error)"=w600) -> ("Daq config Out"=w601:T4, "State Out"=w597:T9, "error out"=w599:errorcluster)  [unwired: 10 in]
                        }
                        frame True {
                          # "If side change or timeout,\nnext state (end shock)"
                          n323 = call "RandomInt64.vi"("Min"=w607, "Max"=w608) -> ("Random"=w606:i64)  [unwired: 9 in]
                          n324 = call "LOOP_pp3c_NextState.vi"("Reward CR"=w603, "New state countdown (ms)"=w606, "New State"=pp3_CTL_BehavioralState."14 Intertrial Interval", "State In"=w605) -> ("State Out"=w609:T9)  [unwired: 7 in]
                        }
                      }
                      n325 = disable-structure shown="Disabled" {
                        frame Disabled {
                          n326 = Wait Until Next ms Multiple(millisecond multiple=u32 1) -> ()  [unwired: 1 out]
                        }
                        frame Enabled {
                        }
                      }
                    }
                    frame "6 GO Jumped", "10 NOGO Timeout", "12 TEST Jumped", "13 TEST Timeout" {
                      # "Response correct,\ngo to ITI immediately"
                      n327 = disable-structure shown="Disabled" {
                        frame Disabled {
                          n328 = Wait Until Next ms Multiple(millisecond multiple=u32 1) -> ()  [unwired: 1 out]
                        }
                        frame Enabled {
                        }
                      }
                      n329 = call "RandomInt64.vi"("Min"=w622, "Max"=w623) -> ("Random"=w619:i64)  [unwired: 9 in]
                      n330 = call "LOOP_pp3c_NextState.vi"("Reward CR"=w612, "New state countdown (ms)"=w619, "New State"=pp3_CTL_BehavioralState."14 Intertrial Interval", "State In"=w621) -> ("State Out"=w620:T9)  [unwired: 7 in]
                    }
                    frame "14 Intertrial Interval" {
                      n331 = case shown="False" w639 {
                        selector: w639 -> [_ w669]
                        tunnel: [TRUE w669] -> w638
                        tunnel: w637 -> [w646 w666]
                        tunnel: w636 -> [w656 w668]
                        tunnel: [w653 w668] -> w635
                        tunnel: w632 -> [w651 w667]
                        tunnel: [w654 w667] -> w631
                        tunnel: [w655 w665] -> w626
                        tunnel: [w652 w666] -> w628
                        tunnel: w627 -> [w642 w665]
                        frame False {
                          # "Paint done trial in table"
                          # "Update stats/close audio (1st loop only)"
                          n332 = Unbundle By Name(w646) -> ("Curr  tr"=w644:u16, "Prev State"=w647:T10)
                          n333 = call "pp3_updateSessionInfo.vi"("Session info In"=w656, "State In"=w646) -> ("Session info Out"=w653:T12)  [unwired: 9 in]
                          n334 = local write "Session info"(w653) -> ()
                          n335 = call "pp3_DAQ_AudioWaitStop.vi"("State info"=w646, "Daq config In"=w642, "error in (no error)"=w651) -> ("State info out"=w648:T9, "Daq config Out"=w655:T4, "error out"=w654:errorcluster)  [unwired: 10 in]
                          n336 = case shown="Default" w647 {
                            tunnel: [u32 52736 u32 11206570 u32 16731983 u32 16763594 u32 12369084 u32 7171459 u32 16776960] -> w645
                            frame "6 GO Jumped" {
                            }
                            frame "7 GO Timeout" {
                            }
                            frame "9 NOGO Jumped" {
                            }
                            frame "10 NOGO Timeout" {
                            }
                            frame "12 TEST Jumped" {
                            }
                            frame "13 TEST Timeout" {
                            }
                            frame Default {
                            }
                          }
                          n337 = Bundle By Name(cluster=w648, "Tone\nGate"=FALSE ("Tone\nGate"), "State update flag"=TRUE) -> (w652:T9)
                          n338 = control-ref of="Session list display"() -> (w643:refnum<vi>)
                          n339 = call "UTIL_pp2_paintTableElement.vi"("Color Box"=w645, "Numeric"=w644, "Tbl Refnum"=w643) -> ()  [unwired: 9 in]
                        }
                        frame True {
                        }
                      }
                      n340 = Wait Until Next ms Multiple(millisecond multiple=u32 1) -> ()  [unwired: 1 out]
                      n341 = case shown="True" w641 {
                        tunnel: [w670 w677] -> w640
                        tunnel: w628 -> [w670 w671]
                        frame False {
                        }
                        frame True {
                          # "Exit if last trial fin\n15s extra video"
                          n342 = Unbundle By Name(w671) -> ("Curr  tr"=w679:u16, "Total trials memo"=w675:i64)
                          n343 = Increment(x=w679) -> (x+1=w673:u16)
                          n344 = Greater Or Equal?(x=w673, y=w675) -> (x >= y?=w674:bool)
                          n345 = case shown="True" w674 {
                            tunnel: [pp3_CTL_BehavioralState."15 Done" ("New State") pp3_CTL_BehavioralState."2 (Load Trial)" ("New State")] -> w676
                            tunnel: [i64 15000 ("New state countdown (ms)") i64 0 ("New state countdown (ms)")] -> w672
                            frame True {
                            }
                            frame False {
                            }
                          }
                          n346 = Bundle By Name(cluster=w671, "Curr  tr"=w673) -> (w678:T9)
                          n347 = call "LOOP_pp3c_NextState.vi"("New state countdown (ms)"=w672, "New State"=w676, "State In"=w678) -> ("State Out"=w677:T9)  [unwired: 8 in]
                        }
                      }
                    }
                    frame "0 NULL", "15 Done" {
                      # "When \"15 Done\" times out,\nsignal will be sent to exit the \nloop"
                      # "\"0 Null\" Will not happen, added to fix compile error"
                      n348 = Wait Until Next ms Multiple(millisecond multiple=u32 3) -> ()  [unwired: 1 out]
                    }
                  }
                  n349 = local read "stop"() -> (w366:bool)
                  n350 = Or(x=w366, y=w362) -> (x .or. y?=w364:bool)
                  n351 = Or(x="Pause", y=w364) -> (x .or. y?=w363:bool)
                  n352 = And(x=w372, y=w363) -> (x .and. y?=w370:bool)
                }
                n353 = local write "DAQ status variable"(w327) -> ()
                n354 = local write "Loop state"(w334) -> ()
              }
              frame #4 {
                # "Will close log file"
                n355 = flat-sequence {
                  frame #0 {
                    # "This done in \"15 Done\"\nloop instead"
                    n356 = disable-structure shown="Disabled" {
                      frame Disabled {
                        # "Always record at least\n10 extra seconds of video"
                        n357 = Wait (ms)(milliseconds to wait=u32 10000) -> ()  [unwired: 1 out]
                      }
                      frame Enabled {
                      }
                    }
                  }
                  frame #1 {
                    w698 = FALSE
                    # "This will stop webcam recording in\nasynchronous processs"
                    n358 = local read "Loop state"() -> (w699:T9)
                    n359 = Bundle By Name(cluster=w699, "Tone\nGate"=w698, "Punish"=w698, "Current DAQ DO Int"=u16 0, "Webcam recording"=w698) -> (w700:T9)
                    n360 = local write "Loop state"(w700) -> ()
                  }
                }
                n361 = Release Queue(queue=w693, error in (no error)=w694) -> (error out=w695:errorcluster)  [unwired: 1 in, 2 out]
                n362 = local write "Runtime Errors"(w695) -> ()
              }
              frame #5 {
                (unwired) u16 0 ("DAQ Digital In")
                # "Post-behavior UI adjustments"
                n363 = local read "DAQ status variable"() -> (w703:T4)
                n364 = local read "Runtime Errors"() -> (w702:errorcluster)
                n365 = property on="Pause" class="Bool (strict)"("DisabledEnum"=T13."Disabled and Grayed Out" ("Disabled")) -> ()  [unwired: 2 in, 2 out]
                n366 = property on="Trial Types Control" class="TabCtl (strict)"("DisabledEnum"=T13."Enabled" ("Disabled")) -> ()  [unwired: 2 in, 2 out]
                n367 = call "DAQ_pp3d_WriteDO.vi"("error in (no error)"=w702, "Daq config"=w703) -> ("error out"=w701:errorcluster)  [unwired: 8 in, 1 out]
                n368 = local write "Runtime Errors"(w701) -> ()
              }
            }
          }
          event "60 trials": Value Change {
            n369 = event-data() -> ()  [unwired: 1 in, 6 out]
            n370 = local read "Session parameters"() -> (w712:T11)
            n371 = Bundle By Name(cluster=w712, "Habit tr0 (s)"=180, "ITI min\n(s)"=14 ("ITI min\n(s)"), "ITI max\n(s)"=24 ("ITI max\n(s)"), "Stay \n(s)"=5 ("Stay \n(s)")) -> (w711:T11)
            n372 = local write "Session parameters"(w711) -> ()
          }
          event "90 trials": Value Change {
            n373 = event-data() -> ()  [unwired: 1 in, 6 out]
            n374 = local read "Session parameters"() -> (w719:T11)
            n375 = Bundle By Name(cluster=w719, "Habit tr0 (s)"=180, "ITI min\n(s)"=6 ("ITI min\n(s)"), "ITI max\n(s)"=16 ("ITI max\n(s)"), "Stay \n(s)"=3 ("Stay \n(s)")) -> (w718:T11)
            n376 = local write "Session parameters"(w718) -> ()
          }
          event "test trials": Value Change {
            n377 = event-data() -> ()  [unwired: 1 in, 6 out]
            n378 = local read "Session parameters"() -> (w726:T11)
            n379 = Bundle By Name(cluster=w726, "Habit tr0 (s)"=5, "ITI min\n(s)"=5 ("ITI min\n(s)"), "ITI max\n(s)"=5 ("ITI max\n(s)"), "Stay \n(s)"=3 ("Stay \n(s)")) -> (w725:T11)
            n380 = local write "Session parameters"(w725) -> ()
          }
        }
      }
    }
    frame #4 {
      w736 = FALSE ("Webcam on")
      w739 = FALSE
      w735 = T13."Enabled" ("Disabled")
      # "Close task only if video used"
      # "Clean up DAQ"
      # "Stop webcam recording"
      # "Post UI Adjustments"
      n381 = local read "Loop state"() -> (w737:T9)
      n382 = Bundle By Name(cluster=w737, "Webcam on"=w736, "Webcam recording"=w736) -> (w738:T9)
      n383 = local write "Loop state"(w738) -> ()
      n384 = property on="DAQ status variable" class="Clust (strict)"("DisabledEnum"=w735) -> ()  [unwired: 2 in, 2 out]
      n385 = property on="Session List Control" class="TabCtl (strict)"("DisabledEnum"=w735) -> ()  [unwired: 2 in, 2 out]
      n386 = property on="Trial Types Control" class="TabCtl (strict)"("DisabledEnum"=w735) -> ()  [unwired: 2 in, 2 out]
      n387 = property on="Session param (dynamic)" class="Clust (strict)"("DisabledEnum"=w735) -> ()  [unwired: 2 in, 2 out]
      n388 = property on="Loop state" class="Clust (strict)"("DisabledEnum"=w735) -> ()  [unwired: 2 in, 2 out]
      n389 = property on="Session parameters" class="Clust (strict)"("DisabledEnum"=w735) -> ()  [unwired: 2 in, 2 out]
      n390 = property on="Session info" class="Clust (strict)"("DisabledEnum"=w735) -> ()  [unwired: 2 in, 2 out]
      n391 = property on="Session list display" class="Tbl (strict)"("Visible"=TRUE) -> ()  [unwired: 2 in, 2 out]
      n392 = local read "DAQ status variable"() -> (w733:T4)
      n393 = local read "Runtime Errors"() -> (w732:errorcluster)
      n394 = local write "stop"(w739) -> ()
      n395 = local write "Pause"(w739) -> ()
      n396 = call "pp3_DAQclear.vi"("error in (no error)"=w732, "Daq config in"=w733) -> ("error out"=w729:errorcluster, "Daq config out"=w734:T4)  [unwired: 8 in]
      n397 = local write "DAQ status variable"(w734) -> ()
      n398 = case shown="True" w728 {
        tunnel: w731 -> [_ w743]
        tunnel: [w740 w742] -> w730
        tunnel: w729 -> [w740 w741]
        frame False {
        }
        frame True {
          n399 = Close Reference(reference=w743, error in (no error)=w741) -> (error out=w742:errorcluster)
        }
      }
      n400 = local write "Runtime Errors"(w730) -> ()
    }
    frame #5 {
      # "Take screenshot for records"
      n401 = local read "Session parameters"() -> (w750:T11)
      n402 = Unbundle By Name(w750) -> ("Log File Directory"=w751:path)
      n403 = control-ref of="This VI"() -> (w747:refnum<vi>)
      n404 = Format Date/Time String(time format string (%c)="%y%m%d_%H%M%S.pp2ss.png" ("pattern (all files)")) -> (date/time string=w748:string)  [unwired: 2 in]
      n405 = Build Path(base path=w751, name or relative path=w748) -> (appended path=w744:path)
      n406 = invoke class="VI" method="FP.Get Image"(reference=w747, "image depth"=24 ("Image Depth")) -> ("image data"=w745:T15)  [unwired: 4 in, 5 out]
      n407 = call <vilib>:"Write PNG File.vi"("image data"=w745, "path to PNG file"=w744) -> ()  [unwired: 8 in, 2 out]
    }
  }
